vi "Preference_Panel.vi"(0 "Mode":T2) -> ()   [LabVIEW 2014]
uses:
  Anemometry Sub Vis/Controls/Server_Comms.ctl
  Anemometry Sub Vis/Controls/Preference_Mode.ctl
  Anemometry Sub Vis/Controls/EnFlo_Data_Folder_Setup.ctl
  Anemometry Sub Vis/File/Setup_Filetype.ctl
  Anemometry Sub Vis/Controls/Overhead.ctl
  ADAM Client/Sub VIs/ADAM Controls/Ch_description_ADAM.ctl
  ADAM Client/Sub VIs/ADAM Controls/Module_type_ADAM.ctl
  ADAM Client/Sub VIs/ADAM Controls/Function_ADAM.ctl
  ADAM Client/Sub VIs/ADAM Controls/Channel_State.ctl
  ADAM Client/Sub VIs/ADAM Controls/Calib_type_ADAM.ctl
  ADAM Client/Sub VIs/ADAM Controls/Address.ctl
  Anemometry Sub Vis/Globals/Constants_global.vi
  Anemometry Sub Vis/Globals/Preference_global.vi
  Anemometry Sub Vis/Globals/Trav_pos_global.vi
  Anemometry Sub Vis/Acquisition/PWA/PWAtasksGLOBAL.vi
panel:
  in  "Traverse to Traverse Collision Detection":bool
  in  "DataTranslation Device No.":u32=20
  in  "Reset Email Counter":bool
  in  "EnFlo_Data_Folder_Setup":T1="EnFlo_Data on Server"
  in  "Post Processing Machine":bool
  in  "Analogue Device Serial No.":string="1188AB4"
  in  "PWA Device Serial No.":string="1187C98"
  in  "ADAM Setup File":u16(ring) items=["Scani_Valve.xls", "Current_Setup.xls"]
  in  "Default Source Establishment Time (s)":dbl=20.0
  out "This Machine's IP Number":string
  in  "Rig Setup":u16(ring) items=["3_x_2_tunnel", "A_Tunnel", "Adam_Sayer_Desk", "ADAM_Server", "Aero_Tunnel", "Alex_Desktop", "B_Tunnel", "Calibration_Tunnel", "Contact_Conductance", "D_Tunnel", "EnFlo_Tunnel", "Frauke_Desktop", "Fruit_Rig", "iMac_G5_2", "iMacDuo1", "Matteo's_desktop", "Matteo_PC", "Nick_PC-2", "Paul_Desk-Paul_Desk_Machine", "Paul_Hayden-Desk", "Paul_N_Desk_Machine_2", "phtest", "Post_Processing_Machine", "PowerBook_G4_1", "PowerBook_G4_2", "Syn_jet_rig", "Tank", "tdf", "Tom_Desk", "Towing_tank", "--New Rig Setup--"]
  in  "Default Traverse Name":u16(ring) items=["A_Tunnel", "Aero_Laser", "Aero_ThroughWall", "Aero_Tunnel", "Angle_Calibrator", "B_Tunnel", "D_Tunnel", "Dummy_Traverse", "EnFlo_Stack", "EnFlo_Tunnel", "EnFlo_Turntable", "Laser_Meas_Traverse", "mohd_setup", "Paul_Desk_Test", "PIV_Traverse", "--New Traverse Setup--"]
  in  "OK":bool
  in  "% Error From First Calib":dbl=10.0 format="%.1f"
  in  "% Error From Previous Calib":dbl=0.5 format="%.1f"
  out "Templates":path=path "/G4_2_HD/Applications (Mac OS 9)/EnFlo Software/Anemometry/Anemometry Sub Vis/Templates"
  in  "Data Folder":path
  out "EnFlo SW Preferences":path=path "/G4_2_HD/Applications (Mac OS 9)/LabVIEW 5.1/EnFlo SW Preferences"
  in  "Tunnel Speed Control":bool
  in  "SMTP server IP address":string
  in  "Abs Press (mbar)":string="Froude:NPL:Atmos_Press"
  in  "Temperature":string="EnFlo Tun:Inlet Heater:Av Temp"
  in  "Server port number":u32=3363
  in  "Server address":string
  in  "LabVIEW Administrators":string[](array[string])=["", "", "", "", "", "", "", "", "", "", "", "", "", "", "", "", "", "", "", ""]
  in  "Server Comms":T3=enum."Do Not Link To Server"
  # "Server Computer Peferences"
  # "Multi Run Preferences"
  # "Warning Levels for Autocalibration Changes"
  # "Email Peferences"
  # "Deg C"
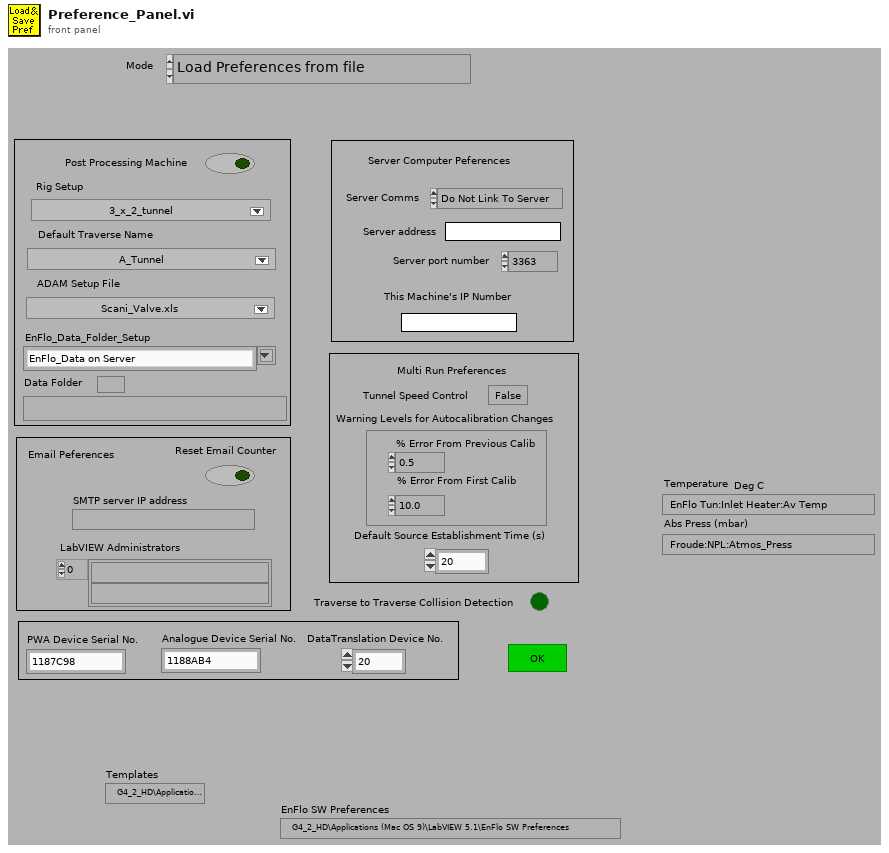
[diagram p1: front panel]
types:
  T1 = typedef "EnFlo_Data_Folder_Setup.ctl" = string
  T2 = typedef "Preference_Mode.ctl" = enum16{"Load Preferences from file", "Save Preferences to file", "Load, Edit then Save"}
  T3 = typedef "Server_Comms.ctl" = enum16{"Server Link Healthy", "Do Not Link To Server"}
  T4 = enum8{"Enabled", "Disabled", "Disabled and Grayed Out"}
  T5 = enum16{"Zero or one", "One", "Zero or more", "One or more"}
  T6 = typedef "Setup_Filetype.ctl" = enum16{"Measurement Setups", "Calibration Setups", "General", "Results File Plotter Setups", "Speed Calib Tweaks"}
  T7 = typedef "Overhead.ctl" = enum16{"Update total times", "Read Current Overhead", "Re Scale totals to 3 hrs", "Initialise totals to 3hr"}
  T8 = typedef "Calib_type_ADAM.ctl" = enum16{"Raw", "Bx + A", "Cx^2 + Bx + A", "Dx^3 + Cx^2 + Bx + A", "In Band", "Hi-Tec Q", "Hi-Tec M_dot", "Text"}
  T9 = typedef "Module_type_ADAM.ctl" = string
  T10 = typedef "Channel_State.ctl" = enum16{"On", "Off", "Always On", "Always Off"}
  T11 = typedef "LVDateTimeRec.ctl" = cluster{"fractional second":dbl, "second":i32, "minute":i32, "hour":i32, "day of month":i32, "month":i32, "year":i32, "day of week":i32, "day of year":i32, "DST":i32}
  T12 = typedef "Ch_description_ADAM.ctl" = cluster{"Ch Name":string, "Type":T9, "Function":T13, "Ch State":T10, "Calibration type":T8, "A":dbl, "B":dbl, "C":dbl, "D":dbl, "Comments":string, "Address":T14, "String":string, "Duty":u16}
  T13 = typedef "Function_ADAM.ctl" = enum16{"Analogue Input", "Digital Input", "Event counter", "Event rate", "Analogue Output", "Digital Output", "Relay Output"}
  T14 = typedef "Address.ctl" = cluster{"Main":i32, "Ch.":i32, "Sub":i32, "Port Name":string}
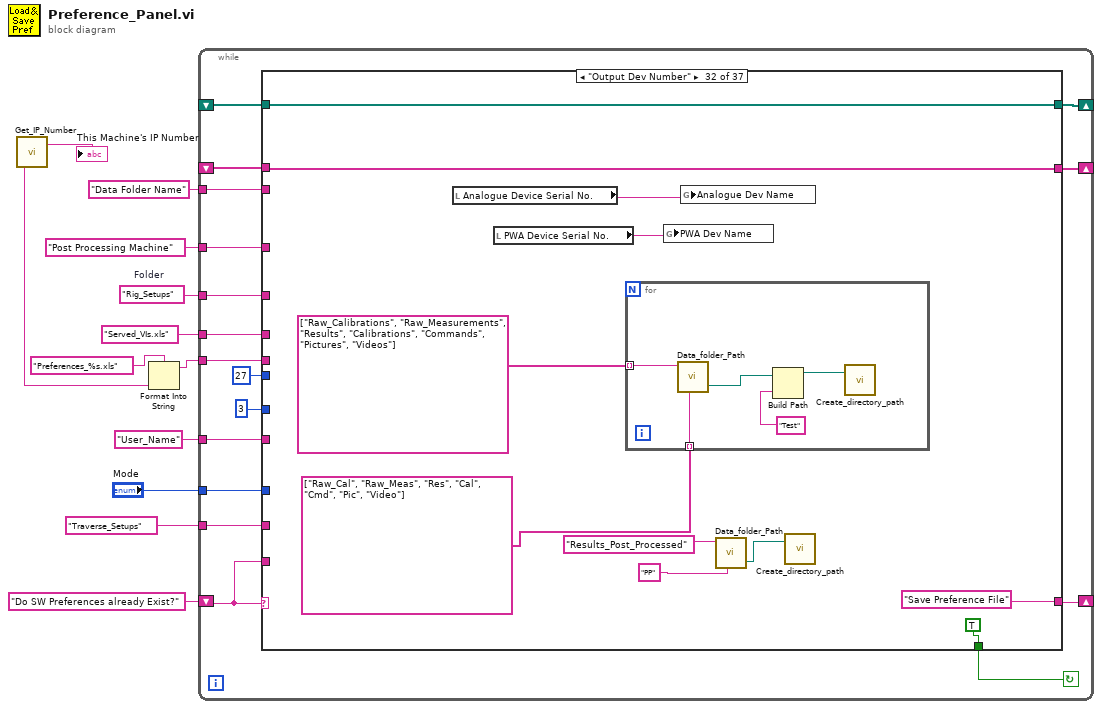
[diagram p0: block diagram]
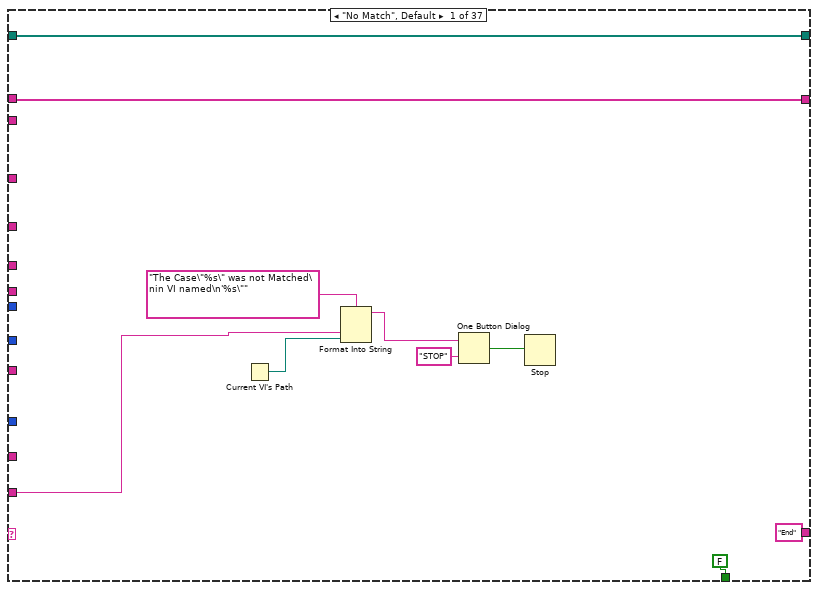
[diagram p2: hidden frame]
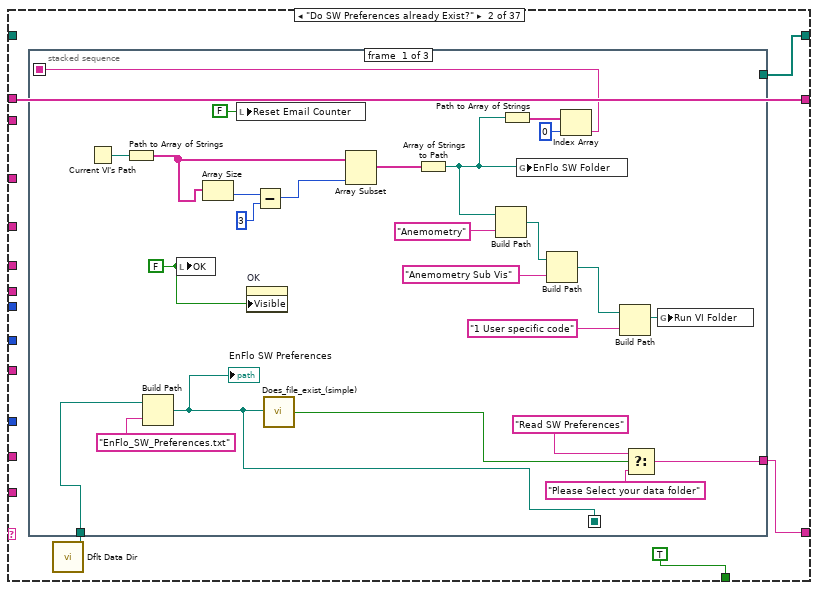
[diagram p3: hidden frame]
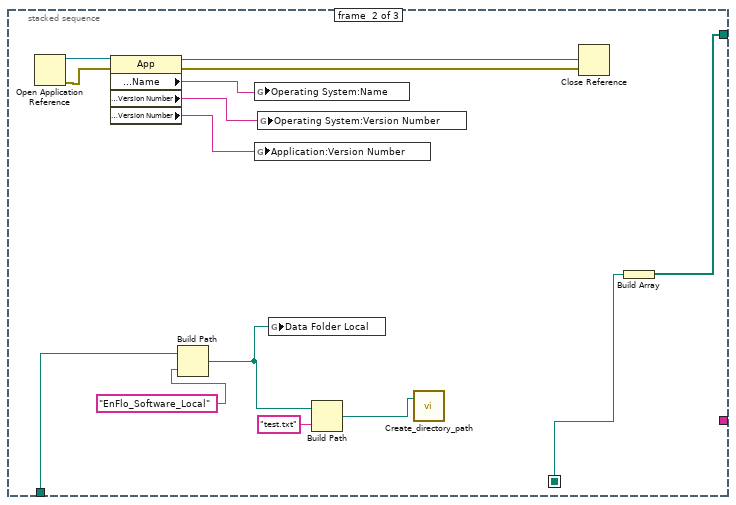
[diagram p4: hidden frame]
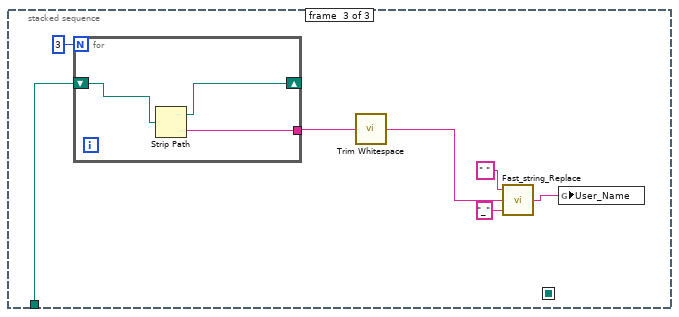
[diagram p5: hidden frame]
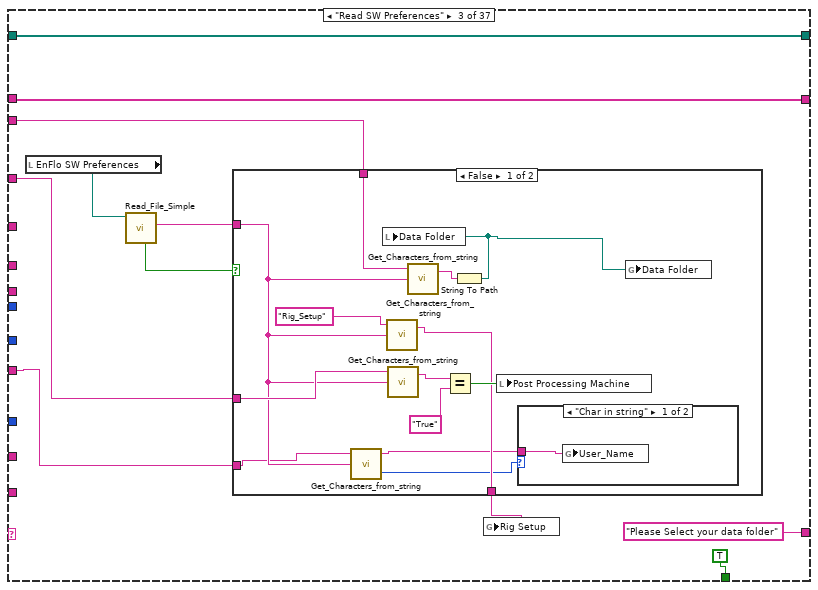
[diagram p6: hidden frame]
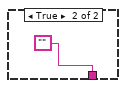
[diagram p8: hidden frame]
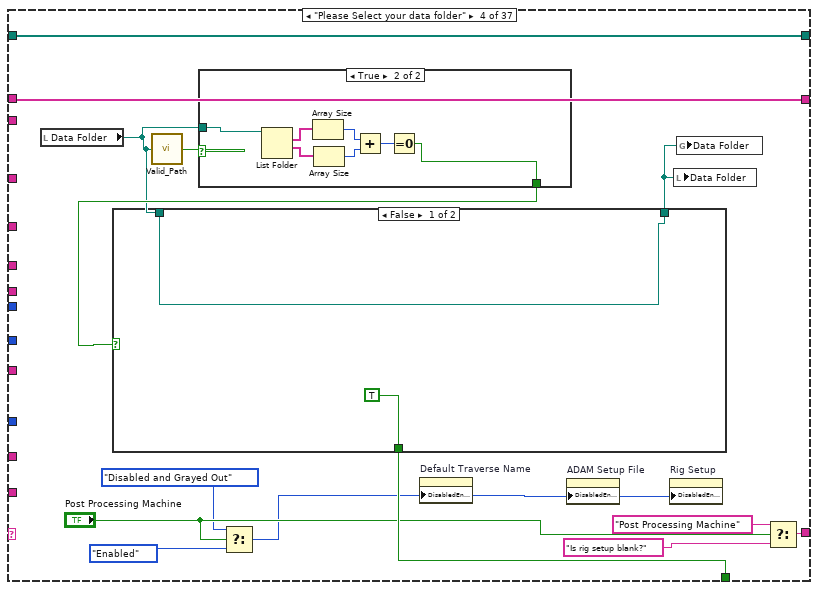
[diagram p9: hidden frame]
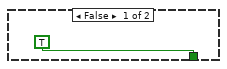
[diagram p10: hidden frame]
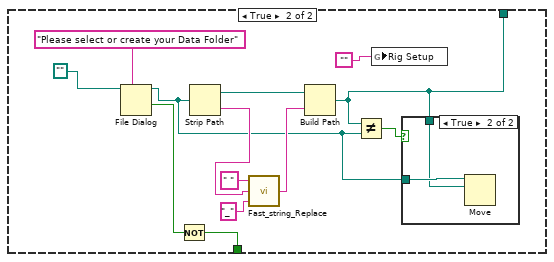
[diagram p11: hidden frame]
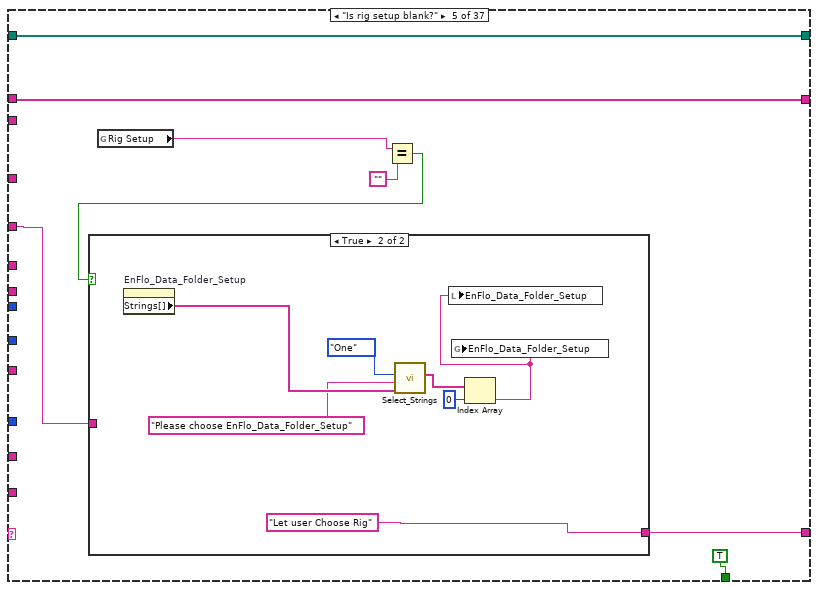
[diagram p13: hidden frame]
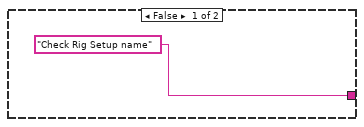
[diagram p14: hidden frame]
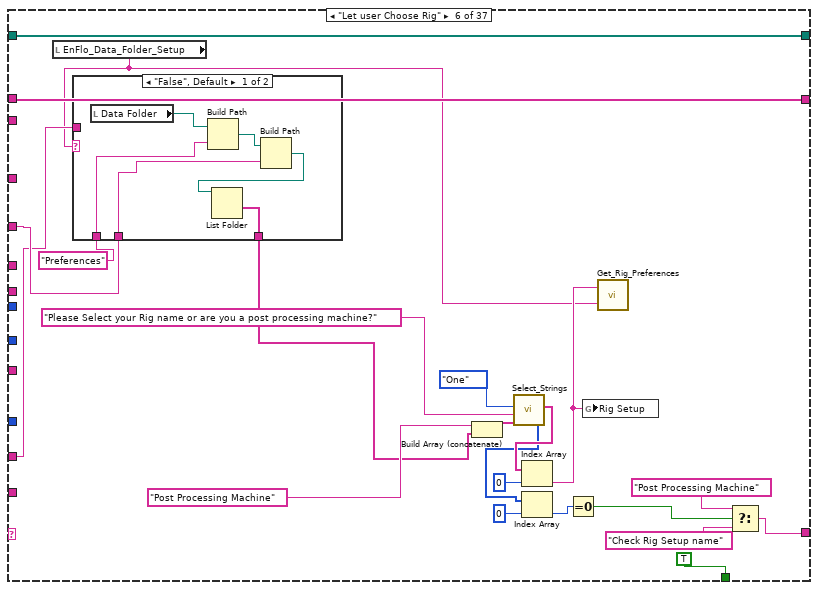
[diagram p15: hidden frame]
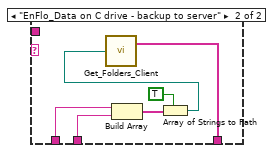
[diagram p16: hidden frame]
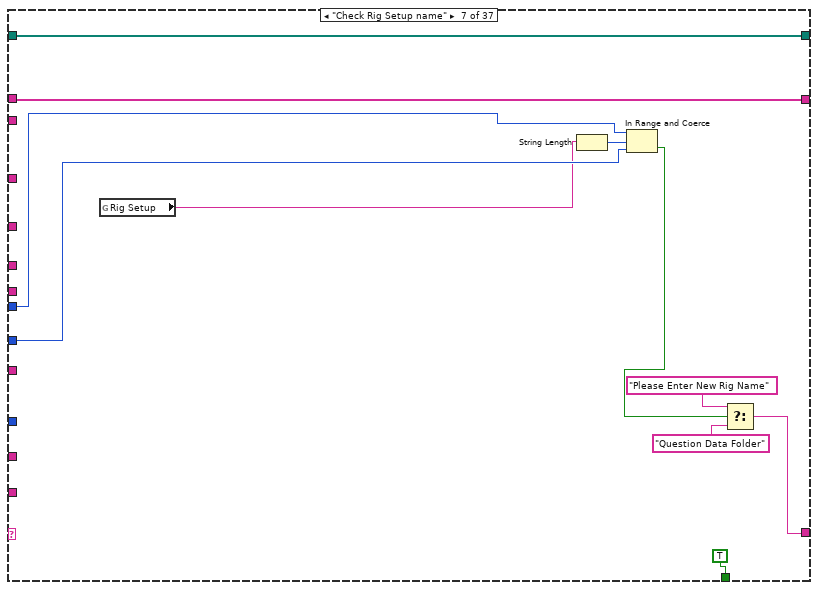
[diagram p17: hidden frame]
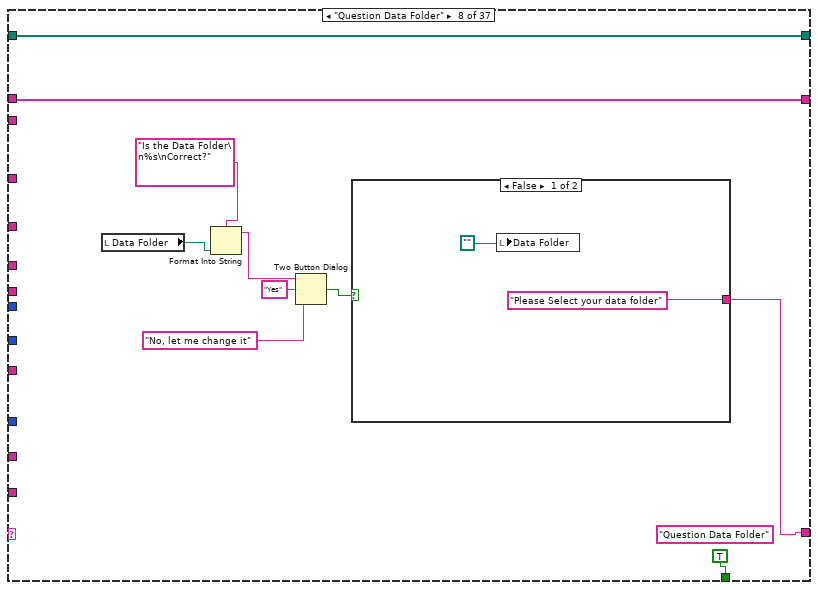
[diagram p18: hidden frame]
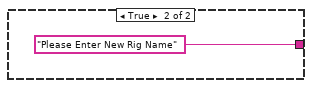
[diagram p19: hidden frame]
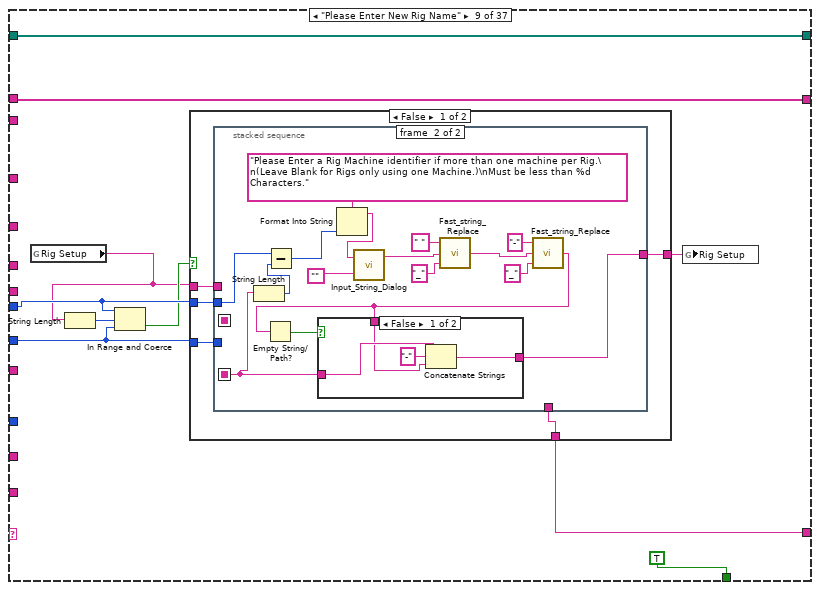
[diagram p20: hidden frame]
diagram:
  w8 = "Rig_Setups"  # Folder
  n1 = call "Get_IP_Number.vi"() -> ("Computer Name"=w3:string, "IP Number"=→"This Machine's IP Number":string)
  n2 = Format Into String(format string="Preferences_%s.xls" ("name or relative path"), w3) -> (resulting string=w1:string)  [unwired: 2 in, 1 out]
  n3 = while {
    shift-left: _ -> [w26]
    shift-right: [w27] -> _
    shift-left: "Do SW Preferences already Exist?" -> [w14]
    shift-right: [w28] -> _
    tunnel: "Mode" -> [w25]
    tunnel: "Data Folder Name" ("Label for characters") -> [w24]
    tunnel: "Served_VIs.xls" ("Substring") -> [w23]
    tunnel: w1 -> [w22]
    tunnel: w8 -> [w19]
    tunnel: "Traverse_Setups" ("name or relative path") -> [w18]
    shift-right: [w17] -> _
    shift-left: _ -> [w16]
    tunnel: "Post Processing Machine" ("Label for characters") -> [w15]
    tunnel: "User_Name" ("Label for characters") -> [w13]
    stop <- w29 continue-if-true
    n4 = case shown="\"Output Dev Number\"" w14 {
      tunnel: [FALSE TRUE TRUE w127 TRUE TRUE TRUE TRUE TRUE TRUE TRUE TRUE TRUE TRUE TRUE TRUE TRUE TRUE TRUE TRUE TRUE TRUE TRUE TRUE TRUE TRUE TRUE TRUE TRUE TRUE TRUE TRUE w882 TRUE TRUE TRUE FALSE] -> w29
      tunnel: ["End" w42 "Please Select your data folder" w124 w159 w192 w209 w220 w239 "Update Constants Global" ("f") "Copy Preferences?" "Copy Preferences?" w368 w385 "Install Preference files" "Install Adam table files" "Install Adam setup files" "Choose ADAM Setup file" "Preference files continued" "Variable Names" w563 w583 "Please Enter new  Traverse Setup" w662 "Create Traverse setup" ("f") "Check file permission status" w759 w790 w810 w830 w846 "Save Preference File" "Save SW Preferences" w957 w971 "Initialise Globals" "End"] -> w28
      tunnel: [w31 w43 w103 w133 w165 w195 w218 w228 w241 w306 w332 w355 w366 w390 w448 w463 w488 w507 w529 w539 w568 w590 w650 w664 w698 w715 w760 w795 w815 w838 w851 w871 w888 w965 w972 w1024 w1083] -> w27
      tunnel: w26 -> [w31 w43 w103 w133 w165 w195 w218 w228 w241 w306 w332 w355 w366 w390 w448 w463 w488 w507 w529 w539 _ w590 w650 w664 w698 w715 w760 w795 w815 w838 w851 w871 w888 w965 w972 w1024 w1083]
      tunnel: w14 -> [w34 _ _ _ _ _ _ _ _ _ _ _ _ _ _ _ _ _ _ _ _ _ _ _ _ _ _ _ _ _ _ _ _ _ _ _ _]
      tunnel: w25 -> [_ _ _ _ _ _ _ _ _ _ _ _ _ _ _ _ _ _ _ _ w562 _ _ _ _ _ w758 _ _ _ _ _ w883 _ _ _ _]
      tunnel: w24 -> [_ _ w100 _ _ _ _ _ _ _ _ _ _ _ _ _ _ _ _ _ _ _ _ _ _ _ _ _ _ _ _ _ _ w956 _ _ _]
      tunnel: w23 -> [_ _ _ _ _ _ _ _ _ _ _ _ _ _ _ w458 _ _ _ _ _ _ _ _ _ _ _ _ _ _ _ _ _ _ _ w1016 _]
      tunnel: w22 -> [_ _ _ _ _ _ _ _ _ _ _ _ w363 w389 _ w454 _ _ _ _ _ w580 _ _ _ _ _ _ _ _ _ _ w879 _ _ _ _]
      tunnel: 3 ("lower limit") -> [_ _ _ _ _ _ w214 _ w238 _ _ _ _ _ _ _ _ _ _ _ _ _ _ w661 _ _ _ _ _ _ _ _ _ _ _ _ _]
      tunnel: 27 ("upper limit") -> [_ _ _ _ _ _ w215 _ w237 _ _ _ _ _ _ _ _ _ _ _ _ _ _ w660 _ _ _ _ _ _ _ _ _ _ _ _ _]
      tunnel: w19 -> [_ _ _ _ w162 w180 _ _ _ w294 w320 _ _ w388 _ _ _ _ _ _ _ _ _ _ _ _ _ _ _ _ _ _ _ _ _ _ _]
      tunnel: w18 -> [_ _ _ _ _ w177 _ _ _ _ _ _ _ _ _ _ _ _ _ _ _ _ w648 _ w685 _ _ _ _ _ _ _ _ _ _ _ _]
      tunnel: [w30 w40 w99 w128 w160 w194 w217 w227 w233 w292 w317 w344 w367 w391 w441 w455 w481 w504 w515 w531 w555 w586 w647 w656 w684 w711 path[] [] w787 w807 w833 w849 w870 w881 w953 w970 w1018 w1081] -> w17
      tunnel: w16 -> [w30 _ w99 w128 w160 w194 w217 w227 w233 w292 w317 w344 w367 w391 w440 w457 w481 w505 w515 w533 w555 w587 w647 w656 w684 w712 w757 w787 w807 w833 w849 w870 w881 w953 w970 w1018 w1081]
      tunnel: w15 -> [_ _ w98 _ _ _ _ _ _ _ _ _ _ _ _ _ _ _ _ _ _ _ _ _ _ _ _ _ _ _ _ _ _ w947 _ _ _]
      tunnel: w13 -> [_ _ w94 _ _ _ _ _ _ _ _ _ _ _ _ _ _ _ _ _ _ _ _ _ _ _ _ _ _ _ _ _ _ w946 _ _ _]
      frame "No Match", Default {
        n5 = Current VI's Path() -> (path=w39:path)
        n6 = Format Into String(format string="The Case\"%s\" was not Matched\nin VI named\n'%s\"" ("Format String"), w34, w39) -> (resulting string=w36:string)  [unwired: 2 in, 1 out]
        n7 = One Button Dialog(message=w36, button name ("OK")="STOP") -> (true=w38:bool)
        n8 = Stop(stop? (T)=w38) -> ()
      }
      frame "Do SW Preferences already Exist?" {
        n9 = call <vilib>:"Dflt Data Dir.vi"() -> ("App:Default Data Directory"=w41:path)
        n10 = stacked-sequence {
          seq-local: [w49 _ _] -> [_ _ _]
          seq-local: [w47 _ _] -> [_ w75 _]
          tunnel: [w53 _ _] -> w42
          tunnel: w41 -> [w48 w73 w89]
          tunnel: [_ w76 _] -> w40
          frame #0 {
            w46 = FALSE ("OK")
            n11 = Current VI's Path() -> (path=w67:path)
            n12 = Path to Array of Strings(0:w67) -> (2:w64:string[])  [unwired: 1 out]
            n13 = Build Path(base path=w48, name or relative path="EnFlo_SW_Preferences.txt") -> (appended path=w47:path)
            "EnFlo SW Preferences" <- w47
            n14 = local write "OK"(w46) -> ()
            n15 = Array Size(array=w64) -> (size(s)=w66:i32)
            n16 = local write "Reset Email Counter"(FALSE ("Reset Email Counter")) -> ()
            n17 = property on="OK" class="Bool (strict)"("Visible"=w46) -> ()  [unwired: 2 in, 2 out]
            n18 = Subtract(x=w66, y=3) -> (x-y=w62:i32)
            n19 = call "Does_file_exist_(simple).vi"("Pathname"=w47) -> ("exists?"=w68:bool)
            n20 = Array Subset(array=w64, length=w62) -> (w63:string[])  [unwired: 1 in]
            n21 = Array of Strings to Path(0:w63) -> (2:w50:path)  [unwired: 1 out]
            n22 = Build Path(base path=w50, name or relative path="Anemometry") -> (appended path=w59:path)
            n23 = Path to Array of Strings(0:w50) -> (2:w51:string[])  [unwired: 1 out]
            n24 = global write "Constants_global.vi" "EnFlo SW Folder"(w50) -> ()
            n25 = Build Path(base path=w59, name or relative path="Anemometry Sub Vis") -> (appended path=w57:path)
            n26 = Index Array(array=w51, index=0) -> (element=w49:string)
            n27 = Build Path(base path=w57, name or relative path="1 User specific code") -> (appended path=w56:path)
            n28 = Select(t="Read SW Preferences", s=w68, f="Please Select your data folder") -> (s? t:f=w53:string)
            n29 = global write "Constants_global.vi" "Run VI Folder"(w56) -> ()
          }
          frame #1 {
            n30 = Open Application Reference() -> (0:w80:errorcluster, 3:w83:refnum<vi>)  [unwired: 1 in, 3 out]
            n31 = property class="App"(reference=w83, error in=w80) -> (reference out=w82:refnum<vi>, error out=w81:errorcluster, "Operating System:Name"=w77:string, "Operating System:Version Number"=w79:string, "Application:Version Number"=w78:string)
            n32 = Build Path(base path=w73, name or relative path="EnFlo_Software_Local" ("element")) -> (appended path=w72:path)
            n33 = global write "Preference_global.vi" "Operating System:Name"(w77) -> ()
            n34 = global write "Preference_global.vi" "Application:Version Number"(w78) -> ()
            n35 = global write "Preference_global.vi" "Operating System:Version Number"(w79) -> ()
            n36 = global write "Constants_global.vi" "Data Folder Local"(w72) -> ()
            n37 = Build Path(base path=w72, name or relative path="test.txt") -> (appended path=w70:path)
            n38 = call "Create_directory_path.vi"("Path name"=w70) -> ()  [unwired: 1 in, 2 out]
            n39 = Close Reference(reference=w82, error in (no error)=w81) -> ()  [unwired: 1 out]
            n40 = Build Array(w75) -> (w76:path[])
          }
          frame #2 {
            n41 = for {
              N: 3 -> [_]
              shift-right: [w93] -> _
              shift-left: w89 -> [w92]
              tunnel: [w91] -> w85
              n42 = Strip Path(path=w92) -> (stripped path=w93:path, name=w91:string)
            }
            n43 = call <vilib>:"Trim Whitespace.vi"("string"=w85) -> ("trimmed string"=w84:string)  [unwired: 1 in]
            n44 = call "Fast_string_Replace.vi"("Replace match with:"="_", "Input String"=w84, "regular expression"=" ") -> ("Output String"=w86:string)  [unwired: 1 in, 1 out]
            n45 = global write "Preference_global.vi" "User_Name"(w86) -> ()
          }
        }
      }
      frame "Read SW Preferences" {
        n46 = local read "EnFlo SW Preferences"() -> (w102:path)
        n47 = call "Read_File_Simple.vi"("Filename"=w102) -> ("Error?"=w96:bool, "string"=w97:string)  [unwired: 2 in, 6 out]
        n48 = case shown="False" w96 {
          tunnel: w100 -> [w116 _]
          tunnel: w98 -> [w113 _]
          tunnel: w97 -> [w108 _]
          tunnel: [w109 ""] -> w95
          tunnel: w94 -> [w107 _]
          frame False {
            n49 = call "Get_Characters_from_string.vi"("Input string"=w108, "Variable name"=w107) -> ("Status"=w106:enum16{"Char in string", "Char not in string"}, "Value"=w105:string)  [unwired: 1 in]
            n50 = call "Get_Characters_from_string.vi"("Input string"=w108, "Variable name"="Rig_Setup" ("Label for characters")) -> ("Value"=w109:string)  [unwired: 1 in, 1 out]
            n51 = call "Get_Characters_from_string.vi"("Input string"=w108, "Variable name"=w113) -> ("Value"=w112:string)  [unwired: 1 in, 1 out]
            n52 = call "Get_Characters_from_string.vi"("Input string"=w108, "Variable name"=w116) -> ("Value"=w117:string)  [unwired: 1 in, 1 out]
            n53 = Equal?(x=w112, y="True") -> (x = y?=w110:bool)
            n54 = String To Path(string=w117) -> (path=w115:path)
            n55 = local write "Data Folder"(w115) -> ()
            n56 = local write "Post Processing Machine"(w110) -> ()
            n57 = case shown="\"Char in string\"" w106 {
              tunnel: w105 -> [w118 _]
              frame "Char in string" {
                n58 = global write "Preference_global.vi" "User_Name"(w118) -> ()
              }
              frame "Char not in string" {
              }
            }
            n59 = global write "Constants_global.vi" "Data Folder"(w115) -> ()
          }
          frame True {
          }
        }
        n60 = global write "Preference_global.vi" "Rig Setup"(w95) -> ()
      }
      frame "Please Select your data folder" {
        n61 = local read "Data Folder"() -> (w129:path)
        n62 = call "Valid_Path.vi"("Filename"=w129) -> ("Valid Path?"=w131:bool)
        n63 = case shown="True" w131 {
          tunnel: [TRUE ("status") w135] -> w130
          tunnel: w129 -> [_ w141]
          frame False {
          }
          frame True {
            n64 = List Folder(path=w141) -> (filenames=w139:string[], folder names=w140:string[])  [unwired: 1 in, 4 out]
            n65 = Array Size(array=w139) -> (size(s)=w137:i32)
            n66 = Array Size(array=w140) -> (size(s)=w138:i32)
            n67 = Add(x=w137, y=w138) -> (x+y=w136:i32)
            n68 = Equal To 0?(x=w136) -> (x = 0?=w135:bool)
          }
        }
        n69 = case shown="False" w130 {
          tunnel: [w143 w147] -> w132
          tunnel: w129 -> [w143 _]
          tunnel: [TRUE w145] -> w127
          frame False {
          }
          frame True {
            n70 = File Dialog(7:"Please select or create your Data Folder" ("prompt"), 11:path "") -> (1:w146:bool, 3:w148:path)  [unwired: 1 in, 6 out]
            n71 = Not(x=w146) -> (.not. x?=w145:bool)
            n72 = Strip Path(path=w148) -> (stripped path=w152:path, name=w151:string)
            n73 = call "Fast_string_Replace.vi"("Replace match with:"="_", "Input String"=w151, "regular expression"=" ") -> ("Output String"=w150:string)  [unwired: 2 out]
            n74 = Build Path(base path=w152, name or relative path=w150) -> (appended path=w147:path)
            n75 = Not Equal?(x=w147, y=w148) -> (x != y?=w149:bool)
            n76 = global write "Preference_global.vi" "Rig Setup"("") -> ()
            n77 = case shown="True" w149 {
              tunnel: w148 -> [_ w158]
              tunnel: w147 -> [_ w157]
              frame False {
              }
              frame True {
                n78 = Move(source path=w158, 10:w157) -> ()  [unwired: 1 in, 5 out]
              }
            }
          }
        }
        n79 = Select(t=T4."Disabled and Grayed Out" ("Disabled"), s="Post Processing Machine", f=T4."Enabled" ("Disabled")) -> (s? t:f=w120:T4)
        n80 = property on="Default Traverse Name" class="Ring (strict)"("DisabledEnum"=w120) -> ()  [unwired: 2 in, 2 out]
        n81 = property on="ADAM Setup File" class="Ring (strict)"("DisabledEnum"=w120) -> ()  [unwired: 2 in, 2 out]
        n82 = property on="Rig Setup" class="Ring (strict)"("DisabledEnum"=w120) -> ()  [unwired: 2 in, 2 out]
        n83 = local write "Data Folder"(w132) -> ()
        n84 = global write "Constants_global.vi" "Data Folder"(w132) -> ()
        n85 = Select(t="Post Processing Machine", s="Post Processing Machine", f="Is rig setup blank?") -> (s? t:f=w124:string)
      }
      frame "Is rig setup blank?" {
        n86 = global read "Preference_global.vi" "Rig Setup"() -> (w161:string)
        n87 = Equal?(x=w161, y="") -> (x = y?=w163:bool)
        n88 = case shown="True" w163 {
          tunnel: w162 -> [_ _]
          tunnel: ["Check Rig Setup name" ("t") "Let user Choose Rig"] -> w159
          frame False {
          }
          frame True {
            n89 = property on="EnFlo_Data_Folder_Setup" class="CmbBox (strict)"() -> ("Strings[]"=w172:string[])  [unwired: 2 in, 2 out]
            n90 = call "Select_Strings.vi"("Available Ch names"=w172, "Message"="Please choose EnFlo_Data_Folder_Setup", "Selector mode"=T5."One") -> ("Selected Channel Names"=w170:string[])  [unwired: 3 in, 2 out]
            n91 = Index Array(array=w170, index=0) -> (element=w168:string)
            n92 = local write "EnFlo_Data_Folder_Setup"(w168) -> ()
            n93 = global write "Preference_global.vi" "EnFlo_Data_Folder_Setup"(w168) -> ()
          }
        }
      }
      frame "Let user Choose Rig" {
        n94 = local read "EnFlo_Data_Folder_Setup"() -> (w175:T1)
        n95 = case shown="\"False\", Default" w175 {
          tunnel: "Preferences" ("name or relative path") -> [w200 w203]
          tunnel: w180 -> [w199 w208]
          tunnel: [w198 w205] -> w178
          tunnel: w177 -> [_ _]
          frame "False", Default {
            n96 = local read "Data Folder"() -> (w201:path)
            n97 = Build Path(base path=w201, name or relative path=w200) -> (appended path=w202:path)
            n98 = Build Path(base path=w202, name or relative path=w199) -> (appended path=w197:path)
            n99 = List Folder(path=w197) -> (folder names=w198:string[])  [unwired: 1 in, 5 out]
          }
          frame "EnFlo_Data on C drive - backup to server" {
            n100 = Build Array(w203, w208) -> (w207:string[])
            n101 = Array of Strings to Path(0:w207, 1:TRUE ("relative")) -> (2:w204:path)
            n102 = call "Get_Folders_Client.vi"("Relative Path"=w204) -> ("Folder Names"=w205:string[])  [unwired: 1 out]
          }
        }
        n103 = Build Array (concatenate)("Post Processing Machine", w178) -> (w185:string[])
        n104 = call "Select_Strings.vi"("Available Ch names"=w185, "Message"="Please Select your Rig name or are you a post processing machine?", "Selector mode"=T5."One") -> ("Ch Indicies Choosen"=w182:i32[], "Selected Channel Names"=w184:string[])  [unwired: 3 in, 1 out]
        n105 = Index Array(array=w184, index=0) -> (element=w176:string)
        n106 = Index Array(array=w182, index=0) -> (element=w181:i32)
        n107 = Equal To 0?(x=w181) -> (x = 0?=w191:bool)
        n108 = global write "Preference_global.vi" "Rig Setup"(w176) -> ()
        n109 = call "Get_Rig_Preferences.vi"("EnFlo_Data_Folder_Setup"=w175, "Rig Setup"=w176) -> ()  [unwired: 1 in]
        n110 = Select(t="Post Processing Machine", s=w191, f="Check Rig Setup name") -> (s? t:f=w192:string)
      }
      frame "Check Rig Setup name" {
        n111 = global read "Preference_global.vi" "Rig Setup"() -> (w210:string)
        n112 = String Length(string=w210) -> (length=w216:i32)
        n113 = In Range and Coerce(upper limit=w215, x=w216, lower limit=w214) -> (In Range?=w213:bool)  [unwired: 1 out]
        n114 = Select(t="Please Enter New Rig Name", s=w213, f="Question Data Folder") -> (s? t:f=w209:string)
      }
      frame "Question Data Folder" {
        (unwired) "Question Data Folder"
        n115 = local read "Data Folder"() -> (w226:path)
        n116 = Format Into String(format string="Is the Data Folder\n%s\nCorrect?" ("message"), w226) -> (resulting string=w224:string)  [unwired: 2 in, 1 out]
        n117 = Two Button Dialog(message=w224, 1:"No, let me change it" ("F button name (\"Cancel\")"), 2:"Yes" ("T button name (\"OK\")")) -> (T button?=w221:bool)
        n118 = case shown="False" w221 {
          tunnel: ["Please Select your data folder" "Please Enter New Rig Name"] -> w220
          frame False {
            n119 = local write "Data Folder"(path "") -> ()
          }
          frame True {
          }
        }
      }
      frame "Please Enter New Rig Name" {
        n120 = global read "Preference_global.vi" "Rig Setup"() -> (w235:string)
        n121 = String Length(string=w235) -> (length=w240:i32)
        n122 = In Range and Coerce(upper limit=w237, x=w240, lower limit=w238) -> (In Range?=w236:bool)  [unwired: 1 out]
        n123 = case shown="False" w236 {
          tunnel: w235 -> [w247 w290]
          tunnel: [w243 "Update Rig setup menu ring"] -> w239
          tunnel: [w244 w290] -> w234
          tunnel: w238 -> [w246 _]
          tunnel: w237 -> [w245 _]
          frame False {
            n124 = stacked-sequence {
              seq-local: [w248 _] -> [_ w273]
              seq-local: [w255 _] -> [_ _]
              tunnel: w247 -> [w257 _]
              tunnel: w246 -> [w268 _]
              tunnel: w245 -> [w254 w271]
              tunnel: [_ w276] -> w244
              tunnel: [w260 _] -> w243
              frame #0 {
                n125 = Match Pattern(string=w257, regular expression="-") -> (before substring=w256:string, after substring=w255:string)  [unwired: 3 out]
                n126 = String Length(string=w255) -> (length=w253:i32)
                n127 = Subtract(x=w254, y=w253) -> (x-y=w252:i32)
                n128 = Format Into String(format string="Please Enter a Rig Name.\n It must be between %d and %d Characters" ("Message to user"), w268, w252) -> (resulting string=w267:string)  [unwired: 2 in, 1 out]
                n129 = call "Input_String_Dialog.vi"("Value"=w256, "Message to user"=w267) -> ("Ok Out"=w263:bool, "Output string"=w264:string)
                n130 = call "Fast_string_Replace.vi"("Replace match with:"="_", "Input String"=w264, "regular expression"=" ") -> ("Output String"=w249:string)  [unwired: 2 out]
                n131 = Select(t="Please Enter New Rig Name", s=w263, f="Save Preference File") -> (s? t:f=w260:string)
                n132 = call "Fast_string_Replace.vi"("Replace match with:"="_", "Input String"=w249, "regular expression"="-") -> ("Output String"=w248:string)  [unwired: 2 out]
              }
              frame #1 {
                n133 = String Length(string=w273) -> (length=w272:i32)
                n134 = Subtract(x=w271, y=w272) -> (x-y=w270:i32)
                n135 = Format Into String(format string="Please Enter a Rig Machine identifier if more than one machine per Rig.\n(Leave Blank for Rigs only using one Machine.)\nMust be less than %d Characters." ("Message to user"), w270) -> (resulting string=w269:string)  [unwired: 2 in, 1 out]
                n136 = call "Input_String_Dialog.vi"("Value"="", "Message to user"=w269) -> ("Output string"=w282:string)  [unwired: 1 out]
                n137 = call "Fast_string_Replace.vi"("Replace match with:"="_", "Input String"=w282, "regular expression"=" ") -> ("Output String"=w278:string)  [unwired: 2 out]
                n138 = call "Fast_string_Replace.vi"("Replace match with:"="_", "Input String"=w278, "regular expression"="-") -> ("Output String"=w275:string)  [unwired: 2 out]
                n139 = Empty String/Path?(string/path=w275) -> (empty?=w277:bool)
                n140 = case shown="False" w277 {
                  tunnel: [w285 w289] -> w276
                  tunnel: w273 -> [w288 w289]
                  tunnel: w275 -> [w286 _]
                  frame False {
                    n141 = Concatenate Strings(w288, "-" ("string"), w286) -> (w285:string)
                  }
                  frame True {
                  }
                }
              }
            }
          }
          frame True {
          }
        }
        n142 = global write "Preference_global.vi" "Rig Setup"(w234) -> ()
      }
      frame "Update Rig setup menu ring" {
        n143 = local read "Data Folder"() -> (w297:path)
        n144 = Build Path(base path=w297, name or relative path="Preferences") -> (appended path=w296:path)
        n145 = global read "Preference_global.vi" "Rig Setup"() -> (w303:string)
        n146 = Build Path(base path=w296, name or relative path=w294) -> (appended path=w295:path)
        n147 = List Folder(path=w295) -> (folder names=w293:string[])  [unwired: 1 in, 5 out]
        n148 = Build Array (concatenate)(w293, "--New Rig Setup--") -> (w299:string[])
        n149 = Search 1D Array(1D array=w299, element=w303) -> (index of element=w302:i32)  [unwired: 1 out]
        n150 = case shown="-1" w302 {
          tunnel: [w309 0] -> w305
          tunnel: w299 -> [w308 w312]
          tunnel: w303 -> [_ w311]
          tunnel: w302 -> [w309 _]
          tunnel: [w308 w310] -> w301
          frame 0, Default {
          }
          frame -1 {
            n151 = Build Array (concatenate)(w311, w312) -> (w310:string[])
          }
        }
        n152 = local write "Rig Setup"(w305) -> ()
        n153 = property on="Rig Setup" class="Ring (strict)"("Strings []"=w301) -> ()  [unwired: 2 in, 2 out]
      }
      frame "Update Constants Global" {
        n154 = global read "Preference_global.vi" "Rig Setup"() -> (w319:string)
        n155 = global read "Constants_global.vi" "Data Folder"() -> (w318:path)
        n156 = Build Path(base path=w318, name or relative path="Preferences") -> (appended path=w321:path)
        n157 = Build Path(base path=w321, name or relative path=w320) -> (appended path=w322:path)
        n158 = Build Path(base path=w322, name or relative path=w319) -> (appended path=w314:path)
        n159 = Build Path(base path=w314, name or relative path="ADAM table") -> (appended path=w327:path)
        n160 = Build Path(base path=w314, name or relative path="Serial") -> (appended path=w326:path)
        n161 = Build Path(base path=w314, name or relative path="All_Users") -> (appended path=w315:path)
        n162 = Build Path(base path=w321, name or relative path="Traverse_Setups") -> (appended path=w325:path)
        n163 = global write "Constants_global.vi" "ADAM setups folder"(w327) -> ()
        n164 = global write "Constants_global.vi" "Serial setups folder"(w326) -> ()
        n165 = global write "Constants_global.vi" "All_Users"(w315) -> ()
        n166 = global write "Constants_global.vi" "Traverse folder"(w325) -> ()
        n167 = Build Array(w327, w326, w315, w325) -> (w324:path[])
        n168 = for {
          tunnel: w324 -> [w336] mode=indexing
          n169 = Build Path(base path=w336, name or relative path="Test") -> (appended path=w334:path)
          n170 = call "Create_directory_path.vi"("Path name"=w334) -> ()  [unwired: 1 in, 2 out]
        }
      }
      frame "Post Processing Machine" {
        n171 = global read "Constants_global.vi" "Data Folder Local"() -> (w343:path)
        n172 = global read "Preference_global.vi" "User_Name"() -> (w338:string)
        n173 = Build Path(base path=w343, name or relative path="Preferences") -> (appended path=w345:path)
        n174 = Build Path(base path=w345, name or relative path=w338) -> (appended path=w339:path)
        n175 = Build Path(base path=w339, name or relative path="ADAM table") -> (appended path=w350:path)
        n176 = Build Path(base path=w339, name or relative path="Serial") -> (appended path=w349:path)
        n177 = Build Path(base path=w339, name or relative path="All_Users") -> (appended path=w340:path)
        n178 = Build Path(base path=w345, name or relative path="Traverse_Setups") -> (appended path=w348:path)
        n179 = local write "Post Processing Machine"(TRUE ("Post Processing Machine")) -> ()
        n180 = global write "Constants_global.vi" "ADAM setups folder"(w350) -> ()
        n181 = global write "Constants_global.vi" "Serial setups folder"(w349) -> ()
        n182 = global write "Constants_global.vi" "All_Users"(w340) -> ()
        n183 = global write "Constants_global.vi" "Traverse folder"(w348) -> ()
        n184 = Build Array(w350, w349, w340, w348) -> (w347:path[])
        n185 = for {
          tunnel: w347 -> [w359] mode=indexing
          n186 = Build Path(base path=w359, name or relative path="Test") -> (appended path=w357:path)
          n187 = call "Create_directory_path.vi"("Path name"=w357) -> ()  [unwired: 1 in, 2 out]
        }
        n188 = global write "Preference_global.vi" "Rig Setup"("Post_Processing_Machine" ("Rig Setup")) -> ()
      }
      frame "Copy Preferences?" {
        n189 = call "Setup_Filepath.vi"("Setup File Type"=Setup_Filetype."General", "Filename in"=w363) -> ("Filename Out"=w362:path)  [unwired: 1 out]
        n190 = call <vilib>:"Check if File or Folder Exists.vi"("path"=w362) -> ("file or folder exists?"=w361:bool)  [unwired: 1 in, 9 out]
        n191 = case shown="False" w361 {
          tunnel: w362 -> [w374 _]
          tunnel: [w372 TRUE ("file or folder exists?")] -> w360
          frame False {
            n192 = Strip Path(path=w374) -> (stripped path=w377:path)  [unwired: 1 out]
            n193 = Build Path(base path=w377, name or relative path="Preferences.xls") -> (appended path=w376:path)
            n194 = Move(source path=w376, 10:w374) -> (3:w373:path)  [unwired: 3 in, 2 out]
            n195 = call <vilib>:"Check if File or Folder Exists.vi"("path"=w373) -> ("file or folder exists?"=w372:bool)  [unwired: 1 in, 9 out]
          }
          frame True {
          }
        }
        n196 = case shown="False" w360 {
          tunnel: [w379 TRUE ("Error?")] -> w365
          frame False {
            n197 = global read "Constants_global.vi" "All_Users"() -> (w381:path)
            n198 = Build Path(base path=w381, name or relative path="Current_Username") -> (appended path=w382:path)
            n199 = call "Read_File_Simple.vi"("Filename"=w382) -> ("Error?"=w379:bool)  [unwired: 4 in, 5 out]
          }
          frame True {
          }
        }
        n200 = Select(t="Install Generic Meas Setup file", s=w365, f="Copy from last user") -> (s? t:f=w368:string)
      }
      frame "Copy from last user" {
        n201 = stacked-sequence {
          seq-local: [w402 _ _ _] -> [_ w412 w421 w433]
          seq-local: [_ w407 _ _] -> [_ _ _ w427]
          seq-local: [_ _ w416 _] -> [_ _ _ w426]
          tunnel: w389 -> [_ w410 _ _]
          tunnel: w388 -> [_ _ _ _]
          tunnel: [_ _ _ w425] -> w387
          frame #0 {
            n202 = global read "Constants_global.vi" "All_Users"() -> (w406:path)
            n203 = Seconds To Date/Time() -> (date time rec=w397:T11)  [unwired: 2 out]
            n204 = Unbundle By Name(w397) -> ("year"=w398:i32)
            n205 = global read "Preference_global.vi" "Rig Setup"() -> (w395:string)
            n206 = Build Path(base path=w406, name or relative path="Current_Username") -> (appended path=w404:path)
            n207 = Number To Decimal String(number=w398) -> (decimal integer string=w396:string)  [unwired: 1 out]
            n208 = global read "Constants_global.vi" "Data Folder"() -> (w401:path)
            n209 = call "Read_File_Simple.vi"("Filename"=w404) -> ("string"=w394:string)  [unwired: 4 in, 5 out]
            n210 = Build Path(base path=w401, name or relative path=w396) -> (appended path=w400:path)
            n211 = Build Path(base path=w400, name or relative path=w395) -> (appended path=w399:path)
            n212 = Build Path(base path=w399, name or relative path=w394) -> (appended path=w403:path)
            n213 = Build Path(base path=w403, name or relative path="Preferences") -> (appended path=w402:path)
          }
          frame #1 {
            n214 = call "Setup_Filepath.vi"("Setup File Type"=Setup_Filetype."General", "Filename in"=w410) -> ("Filename Out"=w409:path)  [unwired: 1 out]
            n215 = Build Path(base path=w412, name or relative path="General") -> (appended path=w414:path)
            n216 = Build Path(base path=w414, name or relative path=w410) -> (appended path=w413:path)
            n217 = Copy(10:w409, 11:w413) -> (0:w408:errorcluster)  [unwired: 3 in, 2 out]
            n218 = Unbundle By Name(w408) -> ("status"=w407:bool)
          }
          frame #2 {
            w419 = "Current_Setup.xls"
            n219 = Build Path(base path=w421, name or relative path="Meas Setups") -> (appended path=w423:path)
            n220 = Build Path(base path=w423, name or relative path=w419) -> (appended path=w422:path)
            n221 = call "Setup_Filepath.vi"("Setup File Type"=Setup_Filetype."Measurement Setups", "Filename in"=w419) -> ("Filename Out"=w418:path)  [unwired: 1 out]
            n222 = Copy(10:w418, 11:w422) -> (0:w417:errorcluster)  [unwired: 3 in, 2 out]
            n223 = Unbundle By Name(w417) -> ("status"=w416:bool)
          }
          frame #3 {
            w431 = "Current_Setup.xls"
            n224 = Build Path(base path=w433, name or relative path="Calib Setups") -> (appended path=w435:path)
            n225 = Build Path(base path=w435, name or relative path=w431) -> (appended path=w434:path)
            n226 = call "Setup_Filepath.vi"("Setup File Type"=Setup_Filetype."Calibration Setups", "Filename in"=w431) -> ("Filename Out"=w430:path)  [unwired: 1 out]
            n227 = Copy(10:w430, 11:w434) -> (0:w429:errorcluster)  [unwired: 3 in, 2 out]
            n228 = Unbundle By Name(w429) -> ("status"=w428:bool)
            n229 = Compound Arithmetic op=OR(w428, w427, w426) -> (w425:bool)
          }
        }
        n230 = Select(t="Install Generic Meas Setup file", s=w387, f="Read SW Preferences") -> (s? t:f=w385:string)
      }
      frame "Install Generic Meas Setup file" {
        n231 = global read "Constants_global.vi" "Run VI Folder"() -> (w447:path)
        n232 = Strip Path(path=w447) -> (stripped path=w445:path)  [unwired: 1 out]
        n233 = call "Setup_Filepath.vi"("Setup File Type"=Setup_Filetype."Measurement Setups", "Filename in"="Current_Setup.xls" ("name or relative path")) -> ("Filename Out"=w437:path)  [unwired: 1 out]
        n234 = Build Path(base path=w445, name or relative path="Templates") -> (appended path=w443:path)
        "Templates" <- w443
        n235 = call "Does_file_exist_(simple).vi"("Pathname"=w437) -> ("exists?"=w444:bool)
        n236 = case shown="False" w444 {
          tunnel: w437 -> [w453 _]
          tunnel: w443 -> [w451 _]
          frame False {
            n237 = Build Path(base path=w451, name or relative path="Measurement Setup.xls") -> (appended path=w450:path)
            n238 = Copy(10:w453, 11:w450) -> ()  [unwired: 1 in, 5 out]
          }
          frame True {
          }
        }
        n239 = Build Array (concatenate)(w440, w437) -> (w441:path[])
      }
      frame "Install Preference files" {
        n240 = Build Array(w454, w458, "Month_Names.xls" ("name or relative path"), "LDA_Configuration.xls") -> (w462:string[])
        n241 = for {
          tunnel: w462 -> [w466] mode=indexing
          tunnel: [w465] -> w456 mode=indexing
          n242 = call "Setup_Filepath.vi"("Setup File Type"=Setup_Filetype."General", "Filename in"=w466) -> ("Filename Out"=w465:path)  [unwired: 1 out]
          n243 = call "Does_file_exist_(simple).vi"("Pathname"=w465) -> ("exists?"=w468:bool)
          n244 = case shown="False" w468 {
            tunnel: w465 -> [w472 _]
            tunnel: w466 -> [w469 _]
            frame False {
              n245 = local read "Templates"() -> (w470:path)
              n246 = Build Path(base path=w470, name or relative path=w469) -> (appended path=w471:path)
              n247 = Copy(10:w472, 11:w471) -> ()  [unwired: 1 in, 5 out]
            }
            frame True {
            }
          }
        }
        n248 = Build Array (concatenate)(w457, w456) -> (w455:path[])
      }
      frame "Install Adam table files" {
        w477 = "Current_Setup.xls"
        n249 = global read "Constants_global.vi" "ADAM setups folder"() -> (w479:path)
        n250 = Build Path(base path=w479, name or relative path=w477) -> (appended path=w480:path)
        n251 = Build Path(base path=w479, name or relative path="Setup_Files") -> (appended path=w475:path)
        n252 = Build Array("Hi_Tec_Calibs.xls" ("name or relative path"), "A_Tunnel DB setup.xls" ("Substring"), "EnFlo_Tunnel DB setup.xls", "Aero_Tunnel DB setup.xls" ("name or relative path"), "D_Tunnel DB setup.xls") -> (w487:string[])
        n253 = Build Path(base path=w475, name or relative path=w477) -> (appended path=w474:path)
        n254 = for {
          tunnel: w487 -> [w491] mode=indexing
          tunnel: w479 -> [w492]
          n255 = Build Path(base path=w492, name or relative path=w491) -> (appended path=w490:path)
          n256 = call "Does_file_exist_(simple).vi"("Pathname"=w490) -> ("exists?"=w493:bool)
          n257 = case shown="False" w493 {
            tunnel: w490 -> [w497 _]
            tunnel: w491 -> [w494 _]
            frame False {
              n258 = local read "Templates"() -> (w495:path)
              n259 = Build Path(base path=w495, name or relative path=w494) -> (appended path=w496:path)
              n260 = Copy(10:w497, 11:w496) -> ()  [unwired: 1 in, 5 out]
            }
            frame True {
            }
          }
        }
        n261 = call "Create_directory_path.vi"("Path name"=w474) -> ("Path name Out"=w473:path)  [unwired: 1 in, 1 out]
        n262 = Move(source path=w480, 10:w473) -> ()  [unwired: 1 in, 5 out]
      }
      frame "Install Adam setup files" {
        w501 = "Current_Setup.xls"
        n263 = global read "Constants_global.vi" "ADAM setups folder"() -> (w503:path)
        n264 = Build Path(base path=w503, name or relative path="Setup_Files") -> (appended path=w500:path)
        n265 = Build Path(base path=w500, name or relative path=w501) -> (appended path=w498:path)
        n266 = call "Does_file_exist_(simple).vi"("Pathname"=w498) -> ("exists?"=w499:bool)
        n267 = case shown="False" w499 {
          tunnel: w498 -> [w514 _]
          tunnel: w501 -> [w512 _]
          frame False {
            n268 = local read "Templates"() -> (w513:path)
            n269 = Build Path(base path=w513, name or relative path="ADAM_Setup_files") -> (appended path=w511:path)
            n270 = Build Path(base path=w511, name or relative path=w512) -> (appended path=w510:path)
            n271 = Copy(10:w514, 11:w510) -> ()  [unwired: 1 in, 5 out]
          }
          frame True {
          }
        }
        n272 = Build Array (concatenate)(w505, w498) -> (w504:path[])
      }
      frame "Choose ADAM Setup file" {
        w523 = "Selected_Filename.txt" ("Substring")
        n273 = global read "Constants_global.vi" "ADAM setups folder"() -> (w527:path)
        n274 = Build Path(base path=w527, name or relative path="Setup_Files") -> (appended path=w524:path)
        n275 = Build Path(base path=w524, name or relative path=w523) -> (appended path=w522:path)
        n276 = call "Read_File_Simple.vi"("Filename"=w522) -> ("string"=w520:string)  [unwired: 2 in, 7 out]
        n277 = Build Array(w523) -> (w525:string[])
        n278 = call "List_files_in_order_of_age.vi"("Files to Hide"=w525, "Folder"=w524) -> ("file names"=w521:string[])
        n279 = Search 1D Array(1D array=w521, element=w520) -> (index of element=w517:i32)  [unwired: 1 out]
        n280 = property on="ADAM Setup File" class="Ring (strict)"("Strings []"=w521) -> ()  [unwired: 2 in, 2 out]
        n281 = Less Than 0?(x=w517) -> (x < 0?=w518:bool)
        n282 = Select(t=0, s=w518, f=w517) -> (s? t:f=w516:i32)
        n283 = local write "ADAM Setup File"(w516) -> ()
      }
      frame "Preference files continued" {
        n284 = Build Array("Hot_Wire_Bridges.txt", "Hot_Wire_Probes.txt", "Pressure_Transducers.txt") -> (w534:string[])
        n285 = for {
          tunnel: w534 -> [w542] mode=indexing
          tunnel: [w541] -> w532 mode=indexing
          n286 = call "Setup_Filepath.vi"("Setup File Type"=Setup_Filetype."Calibration Setups", "Filename in"=w542) -> ("Filename Out"=w541:path)  [unwired: 1 out]
          n287 = call "Does_file_exist_(simple).vi"("Pathname"=w541) -> ("exists?"=w544:bool)
          n288 = case shown="False" w544 {
            tunnel: w541 -> [w548 _]
            tunnel: w542 -> [w545 _]
            frame False {
              n289 = local read "Templates"() -> (w546:path)
              n290 = Build Path(base path=w546, name or relative path=w545) -> (appended path=w547:path)
              n291 = Copy(10:w548, 11:w547) -> ()  [unwired: 1 in, 5 out]
            }
            frame True {
            }
          }
        }
        n292 = Build Array (concatenate)(w533, w532) -> (w531:path[])
      }
      frame "Variable Names" {
        n293 = Build Array("Traverse to Traverse Collision Detection", "DataTranslation Device No.", "PWA Device Serial No.", "Analogue Device Serial No.", "Server address", "Server port number", "LabVIEW Administrators", "SMTP server IP address", "Server Comms", "Default Source Establishment Time (s)", "Temperature", "Abs Press (mbar)", "Default Traverse Name", "Tunnel Speed Control", "Current Overhead Factor", "EnFlo_Data_Central_Repository", "Auto Calib Error fr Previous", "Auto Calib Error fr First", "EnFlo_Data_Folder_Setup") -> (w568:string[])
        n294 = case shown="\"Load, Edit then Save\"" w562 {
          tunnel: ["Load From Preference file" w574 "Save Preference File"] -> w563
          frame "Load Preferences from file" {
          }
          frame "Load, Edit then Save" {
            n295 = local read "OK"() -> (w577:bool)
            n296 = Select(t="Save Preference File", s=w577, f="Load From Preference file") -> (s? t:f=w574:string)
          }
          frame "Save Preferences to file" {
          }
        }
      }
      frame "Load From Preference file" {
        n297 = call "Setup_Filepath.vi"("Setup File Type"=Setup_Filetype."General", "Filename in"=w580) -> ("Filename Out"=w579:path)  [unwired: 1 out]
        n298 = call "Read_File_Simple.vi"("Filename"=w579) -> ("string"=w588:string)  [unwired: 2 in, 7 out]
        n299 = for {
          tunnel: w590 -> [w593] mode=indexing
          tunnel: w588 -> [w592]
          w595 = FALSE  # Show Dialog?
          n300 = call "Get_Characters_from_string.vi"("Show Dialog?"=w595, "Input string"=w592, "Variable name"=w593) -> ("Status"=w594:enum16{"Char in string", "Char not in string"}, "Value"=w591:string)
          n301 = case shown="\"Char in string\"" w594 {
            tunnel: w593 -> [w597 _]
            tunnel: w591 -> [w596 _]
            frame "Char in string" {
              n302 = case shown="\"Analogue Device Serial No.\"" w597 {
                tunnel: w597 -> [w599 _ _ _ _ _ _ _ _ _ _ _ _ _ _ _ _ _ _ _]
                tunnel: w596 -> [_ w600 w601 w604 w605 w608 w609 w610 w612 w614 w617 w620 _ w624 w628 w629 w631 w633 w636 w638]
                tunnel: w596 -> [_ _ _ _ _ _ _ _ _ _ _ _ w621 _ _ _ _ _ _ _]
                frame "No Match", Default {
                  n303 = call "Was_string_matched.vi"("Match Error"=TRUE, "Variable name"=w599) -> ()  [unwired: 1 in]
                }
                frame "Server address" {
                  n304 = global write "Preference_global.vi" "Server address"(w600) -> ()
                  n305 = local write "Server address"(w600) -> ()
                }
                frame "EnFlo_Data_Folder_Setup" {
                  n306 = local write "EnFlo_Data_Folder_Setup"(w601) -> ()
                  n307 = global write "Preference_global.vi" "EnFlo_Data_Folder_Setup"(w601) -> ()
                }
                frame "DataTranslation Device No." {
                  n308 = Decimal String To Number(string=w604, default (0L)=u32 0 ("default (0 I32)")) -> (number=w602:u32)  [unwired: 1 in, 1 out]
                  n309 = global write "Preference_global.vi" "DataTranslation Device No."(w602) -> ()
                  n310 = local write "DataTranslation Device No."(w602) -> ()
                }
                frame "Default Traverse Name" {
                  n311 = global write "Trav_pos_global.vi" "Default Traverse Setup"(w605) -> ()
                }
                frame "Server port number" {
                  n312 = Decimal String To Number(string=w608) -> (number=w607:i32)  [unwired: 3 out]
                  n313 = To Unsigned Long Integer(number=w607) -> (unsigned 32bit integer=w606:u32)
                  n314 = local write "Server port number"(w606) -> ()
                  n315 = global write "Preference_global.vi" "Server port number"(w606) -> ()
                }
                frame "Analogue Device Serial No." {
                  n316 = local write "Analogue Device Serial No."(w609) -> ()
                }
                frame "PWA Device Serial No." {
                  n317 = local write "PWA Device Serial No."(w610) -> ()
                }
                frame "Default Source Establishment Time (s)" {
                  n318 = Fract/Exp String To Number(string=w612) -> (number=w611:dbl)  [unwired: 4 out]
                  n319 = global write "Preference_global.vi" "Default Source Establishment Time (s)"(w611) -> ()
                  n320 = local write "Default Source Establishment Time (s)"(w611) -> ()
                }
                frame "Tunnel Speed Control" {
                  n321 = Equal?(x="TRUE", y=w614) -> (x = y?=w613:bool)
                  n322 = local write "Tunnel Speed Control"(w613) -> ()
                  n323 = global write "Preference_global.vi" "Tunnel Speed Control"(w613) -> ()
                }
                frame "Traverse to Traverse Collision Detection" {
                  n324 = Equal?(x="TRUE", y=w617) -> (x = y?=w616:bool)
                  n325 = global write "Preference_global.vi" "Traverse to Traverse Collision Detection"(w616) -> ()
                  n326 = local write "Traverse to Traverse Collision Detection"(w616) -> ()
                }
                frame "LabVIEW Administrators" {
                  n327 = call "Get_array_values_fr_String.vi"("String Value"=w620) -> ("String array"=w619:string[])  [unwired: 1 out]
                  n328 = global write "Preference_global.vi" "LabVIEW Administrators"(w619) -> ()
                  n329 = local write "LabVIEW Administrators"(w619) -> ()
                }
                frame "SMTP server IP address" {
                  n330 = local write "SMTP server IP address"(w621) -> ()
                  n331 = global write "Preference_global.vi" "SMTP server IP address"(w621) -> ()
                }
                frame "Server Comms" {
                  n332 = Equal?(x="TRUE", y=w624) -> (x = y?=w623:bool)
                  n333 = case shown="False" w623 {
                    tunnel: [Server_Comms."Do Not Link To Server" ("Server Comms") Server_Comms."Server Link Healthy" ("Server Comms")] -> w622
                    frame False {
                    }
                    frame True {
                    }
                  }
                  n334 = local write "Server Comms"(w622) -> ()
                  n335 = global write "Preference_global.vi" "Server Comms"(w622) -> ()
                }
                frame "Temperature" {
                  n336 = global write "Preference_global.vi" "Temperature"(w628) -> ()
                  n337 = local write "Temperature"(w628) -> ()
                }
                frame "Abs Press (mbar)" {
                  n338 = global write "Preference_global.vi" "Abs Press (mbar)"(w629) -> ()
                  n339 = local write "Abs Press (mbar)"(w629) -> ()
                }
                frame "EnFlo_Data_Central_Repository" {
                  n340 = String To Path(string=w631) -> (path=w630:path)
                  n341 = global write "Constants_global.vi" "EnFlo_Data_Central_Repository"(w630) -> ()
                }
                frame "Current Overhead Factor" {
                  n342 = Fract/Exp String To Number(string=w633) -> (number=w632:dbl)  [unwired: 4 out]
                  n343 = call "Overhead_Factor.vi"("Current Overhead Factor In"=w632, "Mode"=Overhead."Initialise totals to 3hr") -> ()  [unwired: 2 in, 1 out]
                }
                frame "Auto Calib Error fr Previous" {
                  n344 = Fract/Exp String To Number(string=w636) -> (number=w635:dbl)  [unwired: 4 out]
                  n345 = global write "Preference_global.vi" "% Error From Previous Calib"(w635) -> ()
                  n346 = local write "% Error From Previous Calib"(w635) -> ()
                }
                frame "Auto Calib Error fr First" {
                  n347 = Fract/Exp String To Number(string=w638) -> (number=w637:dbl)  [unwired: 4 out]
                  n348 = global write "Preference_global.vi" "% Error From First Calib"(w637) -> ()
                  n349 = local write "% Error From First Calib"(w637) -> ()
                }
              }
            }
            frame "Char not in string" {
            }
          }
        }
        n350 = local read "Post Processing Machine"() -> (w585:bool)
        n351 = Select(t="Check file permission status", s=w585, f="is traverse setup blank?") -> (s? t:f=w583:string)
        n352 = Build Array (concatenate)(w587, w579) -> (w586:path[])
      }
      frame "is traverse setup blank?" {
        n353 = local read "Data Folder"() -> (w645:path)
        n354 = global read "Trav_pos_global.vi" "Default Traverse Setup"() -> (w639:string)
        n355 = Build Path(base path=w645, name or relative path="Preferences") -> (appended path=w644:path)
        n356 = Build Path(base path=w644, name or relative path=w648) -> (appended path=w643:path)
        n357 = List Folder(path=w643) -> (folder names=w641:string[])  [unwired: 1 in, 5 out]
        n358 = Search 1D Array(1D array=w641, element=w639) -> (index of element=w642:i32)  [unwired: 1 out]
        n359 = case shown="0, Default" w642 {
          tunnel: w641 -> [_ w654]
          tunnel: [w652 w653] -> w640
          tunnel: w639 -> [w652 _]
          frame 0, Default {
          }
          frame -1 {
            n360 = Index Array(array=w654, index=0) -> (element=w653:string)
          }
        }
        n361 = global write "Trav_pos_global.vi" "Default Traverse Setup"(w640) -> ()
      }
      frame "Please Enter new  Traverse Setup" {
        n362 = global read "Trav_pos_global.vi" "Default Traverse Setup"() -> (w658:string)
        n363 = String Length(string=w658) -> (length=w663:i32)
        n364 = In Range and Coerce(upper limit=w660, x=w663, lower limit=w661) -> (In Range?=w659:bool)  [unwired: 1 out]
        n365 = case shown="False" w659 {
          tunnel: w658 -> [w674 w682]
          tunnel: ["Please Enter new  Traverse Setup" "Update Traverse setup menu ring"] -> w662
          tunnel: [w667 w682] -> w657
          tunnel: w661 -> [w671 _]
          tunnel: w660 -> [w670 _]
          frame False {
            n366 = Format Into String(format string="Please Enter a Traverse Setup Name\nIt must be between %d and %d Characters" ("Message to user"), w671, w670) -> (resulting string=w669:string)  [unwired: 2 in, 1 out]
            n367 = call "Input_String_Dialog.vi"("Value"=w674, "Message to user"=w669) -> ("Ok Out"=w666:bool, "Output string"=w668:string)
            n368 = case shown="False" w666 {
              tunnel: w668 -> [_ w679]
              tunnel: [w675 w678] -> w667
              frame False {
                n369 = property on="Default Traverse Name" class="Ring (strict)"() -> ("Strings []"=w676:string[])  [unwired: 2 in, 2 out]
                n370 = Index Array(array=w676, index=0) -> (element=w675:string)
              }
              frame True {
                n371 = call "Fast_string_Replace.vi"("Replace match with:"="_", "Input String"=w679, "regular expression"=" ") -> ("Output String"=w678:string)  [unwired: 2 out]
              }
            }
          }
          frame True {
          }
        }
        n372 = global write "Trav_pos_global.vi" "Default Traverse Setup"(w657) -> ()
      }
      frame "Update Traverse setup menu ring" {
        n373 = global read "Trav_pos_global.vi" "Default Traverse Setup"() -> (w687:string)
        n374 = local read "Data Folder"() -> (w693:path)
        n375 = Build Path(base path=w693, name or relative path="Preferences") -> (appended path=w692:path)
        n376 = Build Path(base path=w692, name or relative path=w685) -> (appended path=w691:path)
        n377 = List Folder(path=w691) -> (folder names=w689:string[])  [unwired: 1 in, 5 out]
        n378 = Build Array (concatenate)(w689, "--New Traverse Setup--") -> (w688:string[])
        n379 = Search 1D Array(1D array=w688, element=w687) -> (index of element=w695:i32)  [unwired: 1 out]
        n380 = case shown="-1" w695 {
          tunnel: [w701 0] -> w697
          tunnel: w688 -> [w700 w704]
          tunnel: w687 -> [_ w703]
          tunnel: w695 -> [w701 _]
          tunnel: [w700 w702] -> w686
          frame 0, Default {
          }
          frame -1 {
            n381 = Build Array (concatenate)(w703, w704) -> (w702:string[])
          }
        }
        n382 = local write "Default Traverse Name"(w697) -> ()
        n383 = property on="Default Traverse Name" class="Ring (strict)"("Strings []"=w686) -> ()  [unwired: 2 in, 2 out]
      }
      frame "Create Traverse setup" {
        n384 = local read "Templates"() -> (w707:path)
        n385 = Build Path(base path=w707, name or relative path="All_Traverses") -> (appended path=w713:path)
        n386 = stacked-sequence {
          seq-local: [w718 _] -> [_ w746]
          seq-local: [w717 _] -> [_ _]
          tunnel: w713 -> [w720 _]
          tunnel: [w723 _] -> w710
          tunnel: [w722 _] -> w709
          tunnel: w707 -> [_ w745]
          tunnel: [_ w743] -> w706
          frame #0 {
            w726 = "Default_Space_file.xls" ("name or relative path")
            w721 = "Traverse_Setup.xls" ("name or relative path")
            n387 = global read "Trav_pos_global.vi" "Default Traverse Setup"() -> (w717:string)
            n388 = global read "Constants_global.vi" "Traverse folder"() -> (w730:path)
            n389 = Build Path(base path=w720, name or relative path=w726) -> (appended path=w724:path)
            n390 = Build Path(base path=w720, name or relative path=w721) -> (appended path=w719:path)
            n391 = Build Path(base path=w730, name or relative path=w717) -> (appended path=w718:path)
            n392 = Build Path(base path=w718, name or relative path="Trav_Space_Files") -> (appended path=w727:path)
            n393 = Build Path(base path=w727, name or relative path=w726) -> (appended path=w723:path)
            n394 = call "Does_file_exist_(simple).vi"("Pathname"=w723) -> ("exists?"=w725:bool)
            n395 = case shown="False" w725 {
              tunnel: w724 -> [w733 _]
              tunnel: w723 -> [w732 _]
              frame False {
                n396 = call "Create_directory_path.vi"("Path name"=w732) -> ("Path name Out"=w731:path)  [unwired: 1 in, 1 out]
                n397 = Copy(10:w731, 11:w733) -> ()  [unwired: 1 in, 5 out]
              }
              frame True {
              }
            }
            n398 = Build Path(base path=w718, name or relative path=w721) -> (appended path=w722:path)
            n399 = call "Does_file_exist_(simple).vi"("Pathname"=w722) -> ("exists?"=w729:bool)
            n400 = case shown="False" w729 {
              tunnel: w719 -> [w742 _]
              tunnel: w722 -> [w738 _]
              tunnel: w717 -> [w741 _]
              frame False {
                w734 = TRUE  # append to file? (new file:F)
                n401 = call "Create_directory_path.vi"("Path name"=w738) -> ("Path name Out"=w737:path)  [unwired: 1 in, 1 out]
                n402 = call "Read_File_Simple.vi"("Filename"=w742) -> ("string"=w740:string)  [unwired: 2 in, 7 out]
                n403 = call "Fast_string_Replace.vi"("Replace match with:"=w741, "Input String"=w740, "regular expression"="A_Tunnel") -> ("Output String"=w736:string)  [unwired: 2 out]
                n404 = call "Write_Characters_To_File.vi"("file path (dialog if empty)"=w737, "advisory dialog? (display:T)"=TRUE, "character string"=w736, "append to file? (new file:F)"=w734) -> ()  [unwired: 1 in, 4 out]
              }
              frame True {
              }
            }
          }
          frame #1 {
            w744 = "Traverse_Preferences.txt" ("name or relative path")
            n405 = Build Path(base path=w746, name or relative path=w744) -> (appended path=w743:path)
            n406 = Build Path(base path=w745, name or relative path=w744) -> (appended path=w747:path)
            n407 = call "Does_file_exist_(simple).vi"("Pathname"=w743) -> ("exists?"=w748:bool)
            n408 = case shown="False" w748 {
              tunnel: w747 -> [w751 _]
              tunnel: w743 -> [w750 _]
              frame False {
                n409 = call "Create_directory_path.vi"("Path name"=w750) -> ("Path name Out"=w749:path)  [unwired: 1 in, 1 out]
                n410 = Copy(10:w749, 11:w751) -> ()  [unwired: 1 in, 5 out]
              }
              frame True {
              }
            }
          }
        }
        n411 = Build Array (concatenate)(w712, w709, w706, w710) -> (w711:path[])
      }
      frame "Check file permission status" {
        n412 = local read "Post Processing Machine"() -> (w752:bool)
        n413 = for {
          tunnel: w757 -> [w771] mode=indexing
          shift-right: [w768] -> w754
          shift-left: "" -> [w769]
          n414 = call "Can_File_be_Editted.vi"("Filename"=w771) -> ("File Permissions OK?"=w772:bool, "Comment String"=w770:string)  [unwired: 2 out]
          n415 = case shown="False" w772 {
            tunnel: w771 -> [w777 _]
            tunnel: w770 -> [w776 _]
            tunnel: w769 -> [w775 w778]
            tunnel: [w774 w778] -> w768
            frame False {
              n416 = Format Into String(format string="\"%s\" %s\n", initial string=w775, w777, w776) -> (resulting string=w774:string)  [unwired: 1 in, 1 out]
            }
            frame True {
            }
          }
        }
        n417 = case shown="\"Load, Edit then Save\"" w758 {
          tunnel: [w780 w784] -> w759
          tunnel: w752 -> [w779 w783]
          frame "Save Preferences to file", Default {
            n418 = Select(t="Save Preference File", s=w779, f="Output Dev Number") -> (s? t:f=w780:string)
          }
          frame "Load, Edit then Save" {
            n419 = Select(t="Data Folder Changed?", s=w783, f="What next1") -> (s? t:f=w784:string)
          }
        }
        n420 = Empty String/Path?(string/path=w754) -> (empty?=w755:bool)
        n421 = case shown="True" w755 {
          tunnel: w754 -> [w767 _]
          frame False {
            n422 = Concatenate Strings("The following file permissions need to be sorted out before the software will run correctly.\n\n" ("string"), w767) -> (w765:string)
            n423 = Two Button Dialog(message=w765, 1:"Continue" ("F button name (\"Cancel\")"), 2:"Abort" ("F button name (\"Cancel\")")) -> (T button?=w762:bool)
            n424 = Stop(stop? (T)=w762) -> ()
          }
          frame True {
          }
        }
      }
      frame "What next1" {
        n425 = property on="Rig Setup" class="Ring (strict)"() -> ("Strings []"=w789:string[])  [unwired: 2 in, 2 out]
        n426 = Array Size(array=w789) -> (size(s)=w793:i32)
        n427 = Decrement(x=w793) -> (x-1=w792:i32)
        n428 = Equal?(x=w792, y="Rig Setup") -> (x = y?=w791:bool)
        n429 = case shown="False" w791 {
          tunnel: [w797 "Please Enter New Rig Name" ("t")] -> w790
          tunnel: w789 -> [w800 _]
          tunnel: "Rig Setup" -> [w799 _]
          frame False {
            n430 = global read "Preference_global.vi" "Rig Setup"() -> (w801:string)
            n431 = Index Array(array=w800, index=w799) -> (element=w796:string)
            n432 = Not Equal?(x=w796, y=w801) -> (x != y?=w798:bool)
            n433 = case shown="False" w798 {
              tunnel: ["What next2" ("f") "Update Rig setup menu ring" ("t")] -> w797
              tunnel: w796 -> [_ w803]
              frame False {
              }
              frame True {
                n434 = global write "Preference_global.vi" "Rig Setup"(w803) -> ()
              }
            }
          }
          frame True {
            n435 = global write "Preference_global.vi" "Rig Setup"("") -> ()
          }
        }
      }
      frame "What next2" {
        n436 = property on="Default Traverse Name" class="Ring (strict)"() -> ("Strings []"=w809:string[])  [unwired: 2 in, 2 out]
        n437 = Array Size(array=w809) -> (size(s)=w813:i32)
        n438 = Decrement(x=w813) -> (x-1=w812:i32)
        n439 = Equal?(x=w812, y="Default Traverse Name") -> (x = y?=w811:bool)
        n440 = case shown="False" w811 {
          tunnel: [w817 "Please Enter new  Traverse Setup" ("t")] -> w810
          tunnel: w809 -> [w821 _]
          tunnel: "Default Traverse Name" -> [w820 _]
          frame False {
            n441 = global read "Trav_pos_global.vi" "Default Traverse Setup"() -> (w819:string)
            n442 = Index Array(array=w821, index=w820) -> (element=w816:string)
            n443 = Not Equal?(x=w816, y=w819) -> (x != y?=w818:bool)
            n444 = case shown="False" w818 {
              tunnel: ["Data Folder Changed?" ("f") "Update Traverse setup menu ring" ("t")] -> w817
              tunnel: w816 -> [_ w823]
              frame False {
              }
              frame True {
                n445 = global write "Trav_pos_global.vi" "Default Traverse Setup"(w823) -> ()
              }
            }
          }
          frame True {
            n446 = global write "Trav_pos_global.vi" "Default Traverse Setup"("") -> ()
          }
        }
      }
      frame "Data Folder Changed?" {
        w829 = "Please Select your data folder"
        n447 = global read "Constants_global.vi" "Data Folder"() -> (w835:path)
        n448 = local read "Data Folder"() -> (w836:path)
        n449 = property on="OK" class="Bool (strict)"("Visible"=TRUE) -> ()  [unwired: 2 in, 2 out]
        n450 = while {
          shift-right: [w845] -> _
          shift-left: _ -> [w844]
          tunnel: [w843] -> w831
          stop <- TRUE stop-if-true
          n451 = local read "Post Processing Machine"() -> (w845:bool)
          n452 = Not Equal?(x=w845, y=w844) -> (x != y?=w843:bool)
        }
        n453 = Not Equal?(x=w835, y=w836) -> (x != y?=w827:bool)
        n454 = Select(t=w829, s=w827, f="Has OK has been pressed?") -> (s? t:f=w828:string)
        n455 = case shown="True" w831 {
          tunnel: [w839 w841] -> w830
          tunnel: w829 -> [_ w841]
          tunnel: w828 -> [w839 _]
          frame False {
          }
          frame True {
            n456 = global write "Preference_global.vi" "Rig Setup"("") -> ()
          }
        }
      }
      frame "Has OK has been pressed?" {
        n457 = flat-sequence {
          tunnel: ["OK"] -> w847
          frame #0 {
            n458 = Wait (ms)(milliseconds to wait=u32 100) -> ()  [unwired: 1 out]
          }
          frame #1 {
          }
        }
        n459 = local read "Post Processing Machine"() -> (w848:bool)
        n460 = case shown="True" w847 {
          tunnel: w848 -> [w853 w859]
          tunnel: [w852 w856] -> w846
          frame False {
            n461 = Select(t="Data Folder Changed?", s=w853, f="What next1") -> (s? t:f=w852:string)
          }
          frame True {
            n462 = Select(t="Save Preference File", s=w859, f="Output Dev Number") -> (s? t:f=w856:string)
          }
        }
      }
      frame "Output Dev Number" {
        n463 = local read "Analogue Device Serial No."() -> (w867:string)
        n464 = local read "PWA Device Serial No."() -> (w868:string)
        n465 = for {
          tunnel: string[] ["Raw_Calibrations", "Raw_Measurements", "Results", "Calibrations", "Commands", "Pictures", "Videos"] -> [w875] mode=indexing
          tunnel: string[] ["Raw_Cal", "Raw_Meas", "Res", "Cal", "Cmd", "Pic", "Video"] -> [w873] mode=indexing
          n466 = call "Data_folder_Path.vi"("Data Type"=w875, "Short_Name"=w873) -> ("Data Folder"=w874:path)  [unwired: 4 in]
          n467 = Build Path(base path=w874, name or relative path="Test" ("Substring")) -> (appended path=w877:path)
          n468 = call "Create_directory_path.vi"("Path name"=w877) -> ()  [unwired: 1 in, 2 out]
        }
        n469 = global write "PWAtasksGLOBAL.vi" "PWA Dev Name"(w868) -> ()
        n470 = global write "PWAtasksGLOBAL.vi" "Analogue Dev Name"(w867) -> ()
        n471 = call "Data_folder_Path.vi"("Data Type"="Results_Post_Processed" ("element"), "Short_Name"="PP" ("ProjectNumberIn")) -> ("Data Folder"=w864:path)  [unwired: 4 in]
        n472 = call "Create_directory_path.vi"("Path name"=w864) -> ()  [unwired: 1 in, 2 out]
      }
      frame "Save Preference File" {
        n473 = call "Date_and_Time_to_string.vi"() -> ("Date and time (spreadsheet)"=w889:string)
        n474 = call "Setup_Filepath.vi"("Setup File Type"=Setup_Filetype."General", "Filename in"=w879) -> ("Filename Out"=w878:path)  [unwired: 1 out]
        n475 = for {
          tunnel: w888 -> [w899] mode=indexing
          shift-right: [w895] -> w887
          shift-left: w889 -> [w897]
          n476 = case shown="\"Analogue Device Serial No.\"" w899 {
            tunnel: w899 -> [w902 _ _ _ _ _ _ _ _ _ _ _ _ _ _ _ _ _ _ _]
            tunnel: ["No Match" "Server address" "EnFlo_Data_Folder_Setup" w906 w908 w910 w914 w918 "SMTP server IP address" "PWA Device Serial No." "Analogue Device Serial No." w923 w924 w926 "Temperature" "Abs Press (mbar)" w931 w936 w939 w942] -> w898
            frame "No Match", Default {
              n477 = call "Was_string_matched.vi"("Match Error"=TRUE, "Variable name"=w902) -> ()  [unwired: 1 in]
            }
            frame "Server address" {
              n478 = global write "Preference_global.vi" "Server address"("Server address") -> ()
            }
            frame "EnFlo_Data_Folder_Setup" {
              n479 = global write "Preference_global.vi" "EnFlo_Data_Folder_Setup"("EnFlo_Data_Folder_Setup") -> ()
            }
            frame "Server port number" {
              n480 = global write "Preference_global.vi" "Server port number"("Server port number") -> ()
              n481 = Number To Decimal String(number="Server port number") -> (decimal integer string=w906:string)  [unwired: 1 out]
            }
            frame "Default Source Establishment Time (s)" {
              n482 = global write "Preference_global.vi" "Default Source Establishment Time (s)"("Default Source Establishment Time (s)") -> ()
              n483 = Number To Decimal String(number="Default Source Establishment Time (s)") -> (decimal integer string=w908:string)  [unwired: 1 out]
            }
            frame "Tunnel Speed Control" {
              n484 = global write "Preference_global.vi" "Tunnel Speed Control"("Tunnel Speed Control") -> ()
              n485 = Select(t="TRUE", s="Tunnel Speed Control", f="FALSE") -> (s? t:f=w910:string)
            }
            frame "Traverse to Traverse Collision Detection" {
              n486 = global write "Preference_global.vi" "Traverse to Traverse Collision Detection"("Traverse to Traverse Collision Detection") -> ()
              n487 = Select(t="TRUE", s="Traverse to Traverse Collision Detection", f="FALSE") -> (s? t:f=w914:string)
            }
            frame "LabVIEW Administrators" {
              n488 = global write "Preference_global.vi" "LabVIEW Administrators"("LabVIEW Administrators") -> ()
              n489 = call "Put_Array_into_String.vi"("String array"="LabVIEW Administrators") -> ("String Value"=w918:string)
            }
            frame "SMTP server IP address" {
              n490 = global write "Preference_global.vi" "SMTP server IP address"("SMTP server IP address") -> ()
            }
            frame "PWA Device Serial No." {
            }
            frame "Analogue Device Serial No." {
            }
            frame "DataTranslation Device No." {
              n491 = global write "Preference_global.vi" "DataTranslation Device No."("DataTranslation Device No.") -> ()
              n492 = Number To Decimal String(number="DataTranslation Device No.") -> (decimal integer string=w923:string)  [unwired: 1 in]
            }
            frame "Default Traverse Name" {
              n493 = global read "Trav_pos_global.vi" "Default Traverse Setup"() -> (w924:string)
            }
            frame "Server Comms" {
              n494 = case shown="\"Server Link Healthy\"" "Server Comms" {
                tunnel: ["TRUE" "FALSE"] -> w926
                frame "Server Link Healthy" {
                }
                frame "Do Not Link To Server" {
                }
              }
              n495 = global write "Preference_global.vi" "Server Comms"("Server Comms") -> ()
            }
            frame "Temperature" {
              n496 = global write "Preference_global.vi" "Temperature"("Temperature") -> ()
            }
            frame "Abs Press (mbar)" {
              n497 = global write "Preference_global.vi" "Abs Press (mbar)"("Abs Press (mbar)") -> ()
            }
            frame "Current Overhead Factor" {
              n498 = call "Overhead_Factor.vi"("Mode"=Overhead."Read Current Overhead") -> ("Current Overhead Factor"=w933:dbl)  [unwired: 3 in]
              n499 = Number To Fractional String(number=w933, precision (6)=i16 4) -> (F-format string=w931:string)  [unwired: 2 out]
            }
            frame "Auto Calib Error fr Previous" {
              n500 = global write "Preference_global.vi" "% Error From Previous Calib"("% Error From Previous Calib") -> ()
              n501 = Number To Fractional String(number="% Error From Previous Calib", precision (6)=i16 2) -> (F-format string=w936:string)  [unwired: 2 out]
            }
            frame "Auto Calib Error fr First" {
              n502 = global write "Preference_global.vi" "% Error From First Calib"("% Error From First Calib") -> ()
              n503 = Number To Fractional String(number="% Error From First Calib", precision (6)=i16 2) -> (F-format string=w939:string)  [unwired: 2 out]
            }
            frame "EnFlo_Data_Central_Repository" {
              n504 = global read "Constants_global.vi" "EnFlo_Data_Central_Repository"() -> (w941:path)
              n505 = Path To String(path=w941) -> (string=w942:string)
            }
          }
          n506 = call "Characters_to_string.vi"("Characters to write"=w898, "Label for characters"=w899) -> ("Output string"=w896:string)
          n507 = Concatenate Strings(w897, w896) -> (w895:string)
        }
        n508 = case shown="\"Load, Edit then Save\"" w883 {
          tunnel: [TRUE TRUE TRUE] -> w882
          frame "Load, Edit then Save" {
            n509 = Current VI's Path() -> (path=w891:path)
            n510 = call "Open_Close_Front_Panel.ph.vi"("Front Panel Window:Open"=FALSE, "VI path"=w891) -> ()  [unwired: 2 out]
          }
          frame "Load Preferences from file" {
          }
          frame "Save Preferences to file" {
          }
        }
        n511 = call "Write_Characters_To_File.vi"("file path (dialog if empty)"=w878, "advisory dialog? (display:T)"=FALSE, "character string"=w887, "append to file? (new file:F)"=FALSE) -> ()  [unwired: 1 in, 4 out]
      }
      frame "Save SW Preferences" {
        w962 = FALSE  # append to file? (new file:F)
        w963 = FALSE  # advisory dialog? (display:T)
        n512 = local read "Post Processing Machine"() -> (w952:bool)
        n513 = global read "Preference_global.vi" "User_Name"() -> (w945:string)
        n514 = Path To String(path="Data Folder") -> (string=w954:string)
        n515 = global read "Preference_global.vi" "Server Comms"() -> (w958:T3)
        n516 = call "Characters_to_string.vi"("Characters to write"=w954, "Label for characters"=w956) -> ("Output string"=w964:string)
        n517 = Select(t="True", s=w952, f="False") -> (s? t:f=w949:string)
        n518 = call "Characters_to_string.vi"("Characters to write"=w945, "Label for characters"=w946) -> ("Output string"=w944:string)
        n519 = call "Characters_to_string.vi"("Characters to write"=w949, "Label for characters"=w947) -> ("Output string"=w948:string)
        n520 = call "Date_and_Time_to_string.vi"() -> ("Date and time (spreadsheet)"=w959:string)
        n521 = case shown="\"Server Link Healthy\"" w958 {
          tunnel: ["Update Served VI file" "Update Local Adam Table"] -> w957
          frame "Server Link Healthy" {
          }
          frame "Do Not Link To Server" {
          }
        }
        n522 = Concatenate Strings(w959, w964, w948, w944) -> (w960:string)
        n523 = local read "EnFlo SW Preferences"() -> (w961:path)
        n524 = call "Write_Characters_To_File.vi"("file path (dialog if empty)"=w961, "advisory dialog? (display:T)"=w963, "character string"=w960, "append to file? (new file:F)"=w962) -> ()  [unwired: 1 in, 4 out]
        n525 = case shown="True" "Reset Email Counter" {
          tunnel: "Reset Email Counter" -> [_ w967]
          frame False {
          }
          frame True {
            n526 = global write "Preference_global.vi" "Unblock Email"(w967) -> ()
          }
        }
      }
      frame "Update Local Adam Table" {
        n527 = stacked-sequence {
          seq-local: [w979 _] -> [_ w993]
          tunnel: ["Update Served VI file" _] -> w971
          frame #0 {
            w979 = T12 {"Ch Name"="", "Type"="", "Function"=enum."Analogue Input", "Ch State"=enum."On", "Calibration type"=enum."Raw", "A"=0.0, "B"=0.0, "C"=0.0, "D"=0.0, "Comments"="", "Address"={"Main"=0, "Ch."=0, "Sub"=0, "Port Name"=""}, "String"="", "Duty"=0} ("Ch Discription")
            n528 = global read "Preference_global.vi" "Abs Press (mbar)"() -> (w976:string)
            n529 = global read "Preference_global.vi" "Temperature"() -> (w977:string)
            n530 = Bundle By Name(cluster=w979, "Type"=T9 "", "Calibration type"=Calib_type_ADAM."Raw", "A"=1.0) -> (w980:T12)
            n531 = Build Array(w977, w976) -> (w975:string[])
            n532 = for {
              tunnel: [w986] -> w978 mode=indexing
              tunnel: w980 -> [w985]
              tunnel: w975 -> [w984] mode=indexing
              n533 = Bundle By Name(cluster=w985, "Ch Name"=w984) -> (w986:T12)
            }
            n534 = call "Update_Ch_Discription_client.vi"("Channels to update In"=w978) -> ()  [unwired: 1 out]
          }
          frame #1 {
            n535 = global read "Preference_global.vi" "Rig Setup"() -> (w988:string)
            n536 = call "Get_Current_Scan_client.vi"() -> ("Ch Description Array"=w994:T12[])  [unwired: 1 in, 3 out]
            n537 = Match Pattern(string=w988, regular expression="-") -> (before substring=w987:string)  [unwired: 4 out]
            n538 = Format Into String(format string="%s Metadata:" ("Format String"), w987) -> (resulting string=w996:string)  [unwired: 2 in, 1 out]
            n539 = Initialize Array(w993, 0 ("dimension size")) -> (w991:T12[])
            n540 = for {
              shift-right: [w1007] -> w990
              shift-left: w991 -> [w1008]
              tunnel: w994 -> [w999] mode=indexing
              tunnel: w996 -> [w1006]
              tunnel: "Metadata:" ("Format String") -> [w1005]
              n541 = Unbundle By Name(w999) -> ("Ch Name"=w998:string)
              n542 = Match Pattern(string=w998, regular expression=w1006) -> (offset past match=w1003:i32)  [unwired: 4 out]
              n543 = Match Pattern(string=w998, regular expression=w1005) -> (offset past match=w1004:i32)  [unwired: 4 out]
              n544 = Greater Or Equal To 0?(x=w1004) -> (x >= 0?=w1001:bool)
              n545 = Less Than 0?(x=w1003) -> (x < 0?=w1002:bool)
              n546 = And(x=w1002, y=w1001) -> (x .and. y?=w1000:bool)
              n547 = case shown="True" w1000 {
                tunnel: w1008 -> [w1009 w1014]
                tunnel: [w1009 w1013] -> w1007
                tunnel: w999 -> [_ w1012]
                frame False {
                }
                frame True {
                  n548 = Bundle By Name(cluster=w1012, "Ch State"=Channel_State."Off") -> (w1010:T12)
                  n549 = Build Array (concatenate)(w1014, w1010) -> (w1013:T12[])
                }
              }
            }
            n550 = call "Update_Ch_Discription_client.vi"("Channels to update In"=w990) -> ()  [unwired: 1 out]
          }
        }
      }
      frame "Update Served VI file" {
        # "Template"
        # "Orig"
        n551 = call "Setup_Filepath.vi"("Setup File Type"=Setup_Filetype."General", "Filename in"=w1016) -> ("Filename Out"=w1015:path)  [unwired: 1 out]
        n552 = Build Array("Served:VI:Name", "Served:VI:Path", "Server:IP Number:& Port No") -> (w1021:string[])
        n553 = stacked-sequence {
          seq-local: [w1026 _ _ _] -> [_ _ w1036 _]
          seq-local: [_ w1033 _ _] -> [_ _ w1037 _]
          seq-local: [_ _ w1038 _] -> [_ _ _ w1063]
          tunnel: w1021 -> [w1028 w1034 _ w1064]
          tunnel: w1015 -> [w1027 _ _ w1065]
          tunnel: w1016 -> [_ w1030 _ _]
          frame #0 {
            n554 = call "Read_Ch_data_file.vi"("Present Channels"=w1028, "Output"=enum16{"All Ch data", "The last few rows"}."All Ch data", "Filename"=w1027) -> ("Channel Values"=w1026:string[][])  [unwired: 2 in, 4 out]
          }
          frame #1 {
            n555 = local read "Templates"() -> (w1032:path)
            n556 = Build Path(base path=w1032, name or relative path=w1030) -> (appended path=w1031:path)
            n557 = call "Read_Ch_data_file.vi"("Present Channels"=w1034, "Output"=enum16{"All Ch data", "The last few rows"}."All Ch data", "Filename"=w1031) -> ("Channel Values"=w1033:string[][])  [unwired: 2 in, 4 out]
          }
          frame #2 {
            n558 = Index Array(array=w1036, index (col)=0 ("Index")) -> (element=w1041:string[])  [unwired: 1 in]
            n559 = To Upper Case(1:w1037) -> (0:w1039:string[][])
            n560 = To Upper Case(1:w1041) -> (0:w1040:string[])
            n561 = for {
              tunnel: w1040 -> [w1044]
              tunnel: w1037 -> [w1049] mode=indexing
              tunnel: w1039 -> [w1043] mode=indexing
              tunnel: [w1046] -> w1038 mode=indexing
              tunnel: w1036 -> [w1045]
              n562 = Index Array(array=w1043, index=0 ("Index")) -> (element=w1047:string)
              n563 = Search 1D Array(1D array=w1044, element=w1047) -> (index of element=w1048:i32)  [unwired: 1 out]
              n564 = case shown="0, Default" w1048 {
                tunnel: w1049 -> [w1058 w1059]
                tunnel: w1048 -> [w1055 _]
                tunnel: [w1051 w1059] -> w1046
                tunnel: w1045 -> [w1056 _]
                frame 0, Default {
                  n565 = Index Array(array=w1056, index (row)=w1055, index (col)=2 ("Index")) -> (element=w1053:string)
                  n566 = Array Subset(array=w1058, length=2) -> (w1052:string[])  [unwired: 1 in]
                  n567 = Build Array (concatenate)(w1052, w1053) -> (w1051:string[])
                }
                frame -1 {
                }
              }
            }
          }
          frame #3 {
            w1060 = FALSE  # Append last row only
            w1061 = FALSE  # Lock File
            w1062 = FALSE  # exists?
            n568 = call "Write_Ch_data_file.vi"("Append last row only"=w1060, "Lock File"=w1061, "exists?"=w1062, "Channel Values"=w1063, "Channel names"=w1064, "Filename"=w1065) -> ()  [unwired: 2 in, 4 out]
          }
        }
      }
      frame "Initialise Globals" {
        w1070 = TRUE  # OK
        w1074 = FALSE  # append to file? (new file:F)
        w1073 = FALSE  # advisory dialog? (display:T)
        n569 = global read "Constants_global.vi" "ADAM setups folder"() -> (w1080:path)
        n570 = global read "Constants_global.vi" "All_Users"() -> (w1069:path)
        n571 = property on="ADAM Setup File" class="Ring (strict)"() -> ("Strings []"=w1075:string[])  [unwired: 2 in, 2 out]
        n572 = Build Path(base path=w1069, name or relative path="Current_Username") -> (appended path=w1067:path)
        n573 = Build Path(base path=w1080, name or relative path="Setup_Files") -> (appended path=w1078:path)
        n574 = global read "Preference_global.vi" "User_Name"() -> (w1066:string)
        n575 = Build Path(base path=w1078, name or relative path="Selected_Filename.txt" ("Substring")) -> (appended path=w1071:path)
        n576 = call "Get_users_email_addresses.vi"("OK"=w1070) -> ()  [unwired: 5 out]
        n577 = Index Array(array=w1075, index="ADAM Setup File") -> (element=w1072:string)
        n578 = call "Write_File_Simple.vi"("character string"=w1066, "file path"=w1067) -> ()  [unwired: 1 in, 2 out]
        n579 = call "Write_Characters_To_File.vi"("file path (dialog if empty)"=w1071, "advisory dialog? (display:T)"=w1073, "character string"=w1072, "append to file? (new file:F)"=w1074) -> ()  [unwired: 1 in, 4 out]
      }
    }
  }
